vi "FPGA_Main_v7.vi"() -> ()   [LabVIEW 2018]
uses:
  <vilib>/Platform/TimedLoop/XDataNode/XDataNode.xnode
  <vilib>/Platform/TimedLoop/XDataNode/nitl_modes.ctl
  <vilib>/Platform/TimedLoop/XDataNode/XDNodeRunTimeDep.lvlib
  <vilib>/Platform/TimedLoop/XDataNode/wakeup.ctl
  <vilib>/Platform/TimedLoop/XDataNode/timing_clust.ctl
  <vilib>/rvi/DataTransferAndStorage/Container/XNode/niFpgaContainer.xnode
  <vilib>/rvi/FIFO/Fifo_Resource/nirvififoEmulationRead.vi
  <vilib>/eio/EIONode/EIONode.xnode
  <vilib>/rvi/eio/common/nirviEmuTemplateMethod_errors.vi
  <vilib>/rvi/DataTransferAndStorage/Register/Emulation/niFpgaRegisterEmulation.vi
  <instrlib>/_niInstr/Basic Elements/v1/FPGA/niInstr Basic Elements v1 FPGA.lvlib
  <vilib>/rvi/FIFO/Fifo_Resource/nirvififoEmulationWrite.vi
  <vilib>/rvi/interface/RandomDataEmulation/nirviRandomDataFpgaReadWriteTemplate.vi
  <instrlib>/_niInstr/Basic Elements/v1/FPGA/Private/Count Down U32.vi
  <instrlib>/_niInstr/Basic Elements/v1/FPGA/Private/Count Up U8.vi
  <vilib>/rvi/Memory/Memory_Emulation/nirvimemoryFastEmulation.vi
  <vilib>/rvi/Memory/Memory_Emulation/nirvimemoryEmulation.vi
  <vilib>/eio/EIOPropertyNode/EIOPropertyNode.xnode
  <vilib>/LabVIEW Targets/FPGA/RIO/BlueMoonOnboardIO/nicrio_cRIO-BlueMoonOnboardAi_TerminalMod.ctl
  <vilib>/rvi/eio/common/nirviEmuTemplatePropertyGet_errors.vi
  <vilib>/rvi/eio/common/nirviEmuTemplatePropertyGet_noerrors.vi
  <vilib>/rvi/eio/common/nirviEmuTemplatePropertySet_errors.vi
  <vilib>/rvi/eio/common/nirviEmuTemplatePropertySet_noerrors.vi
  <vilib>/LabVIEW Targets/FPGA/RIO/BlueMoonOnboardIO/nicrio_cRIO-BlueMoonOnboardAi_VoltageRange.ctl
  <instrlib>/_niInstr/Basic Elements/v1/FPGA/Private/Count Up U32.vi
panel:
  out "AuxArbWfm":u32
  in  "Reset":bool
  out "SubEventCode":u8
  out "Daq.Length?":u32
  in  "Start":bool
  out "RFU64 Ele#":u32
  out "EventCode Ele#":u32
  out "SigI16 Ele#":u32
  out "EventCode":u8
  out "DI":u8
  out "IonGateAGC.Time":u32
  out "IonGateAGC.Value":u64
  out "IonGateAGC.Target*TrialTime":u64
  out "Daq.AqNumber?":u32
  out "Daq.HighestValue_I16":i16
  out "AI.ReadingClocks":u32
  out "LaserTrig.Enable?":bool
  out "Event.Scan?":bool
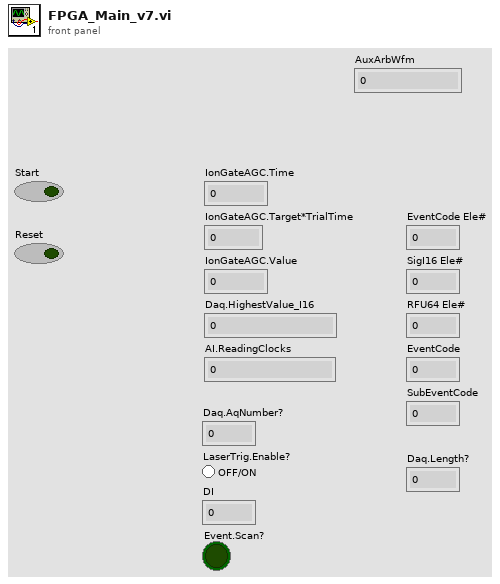
[diagram p1: front panel]
types:
  T1 = typedef "nicrio_cRIO-BlueMoonOnboardAi_VoltageRange.ctl" = u8
  T2 = typedef "nicrio_cRIO-BlueMoonOnboardAi_TerminalMod.ctl" = u8
  T3 = typedef "XDNodeRunTimeDep.lvlib/timing_clust.ctl" = cluster{"Expected End [f-1]":u64, "Actual End [f-1]":u64, "Finished Late? [f-1]":bool, "Expected End [i-1]":u64, "Actual End [i-1]":u64, "Finished Late? [i-1]":bool, "Expected Start [i]":u64, "Actual Start [i]":u64, "Expected Start [f]":u64, "Actual Start [f]":u64, "Source Name":string, "Structure Name":string, "Period":i64, "Deadline":i64, "Offset":i64, "Start":i64, "Priority":i32, "Timeout":i32, "Mode":T4, "Wakeup Reason":T5, "Error":errorcluster, "Source Type":string, "Secondary Source Type":string, "Global End Time":u64, "Global Start Time":u64, "Frame Duration":u64, "Iteration Duration":u64, "Assigned CPU":i32, "I/O Scan Engine Mode":u32}
  T4 = typedef "XDNodeRunTimeDep.lvlib/nitl_modes.ctl" = enum32{"No Change", "Process missed periods, maintain original phase", "Discard missed periods, maintain original phase", "Process missed periods, ignore original phase", "Discard missed periods, ignore original phase"}
  T5 = typedef "XDNodeRunTimeDep.lvlib/wakeup.ctl" = enum32{"Normal", "Aborted", "Asynchronous wakeup", "Timing source error", "Timed loop error", "Timeout"}
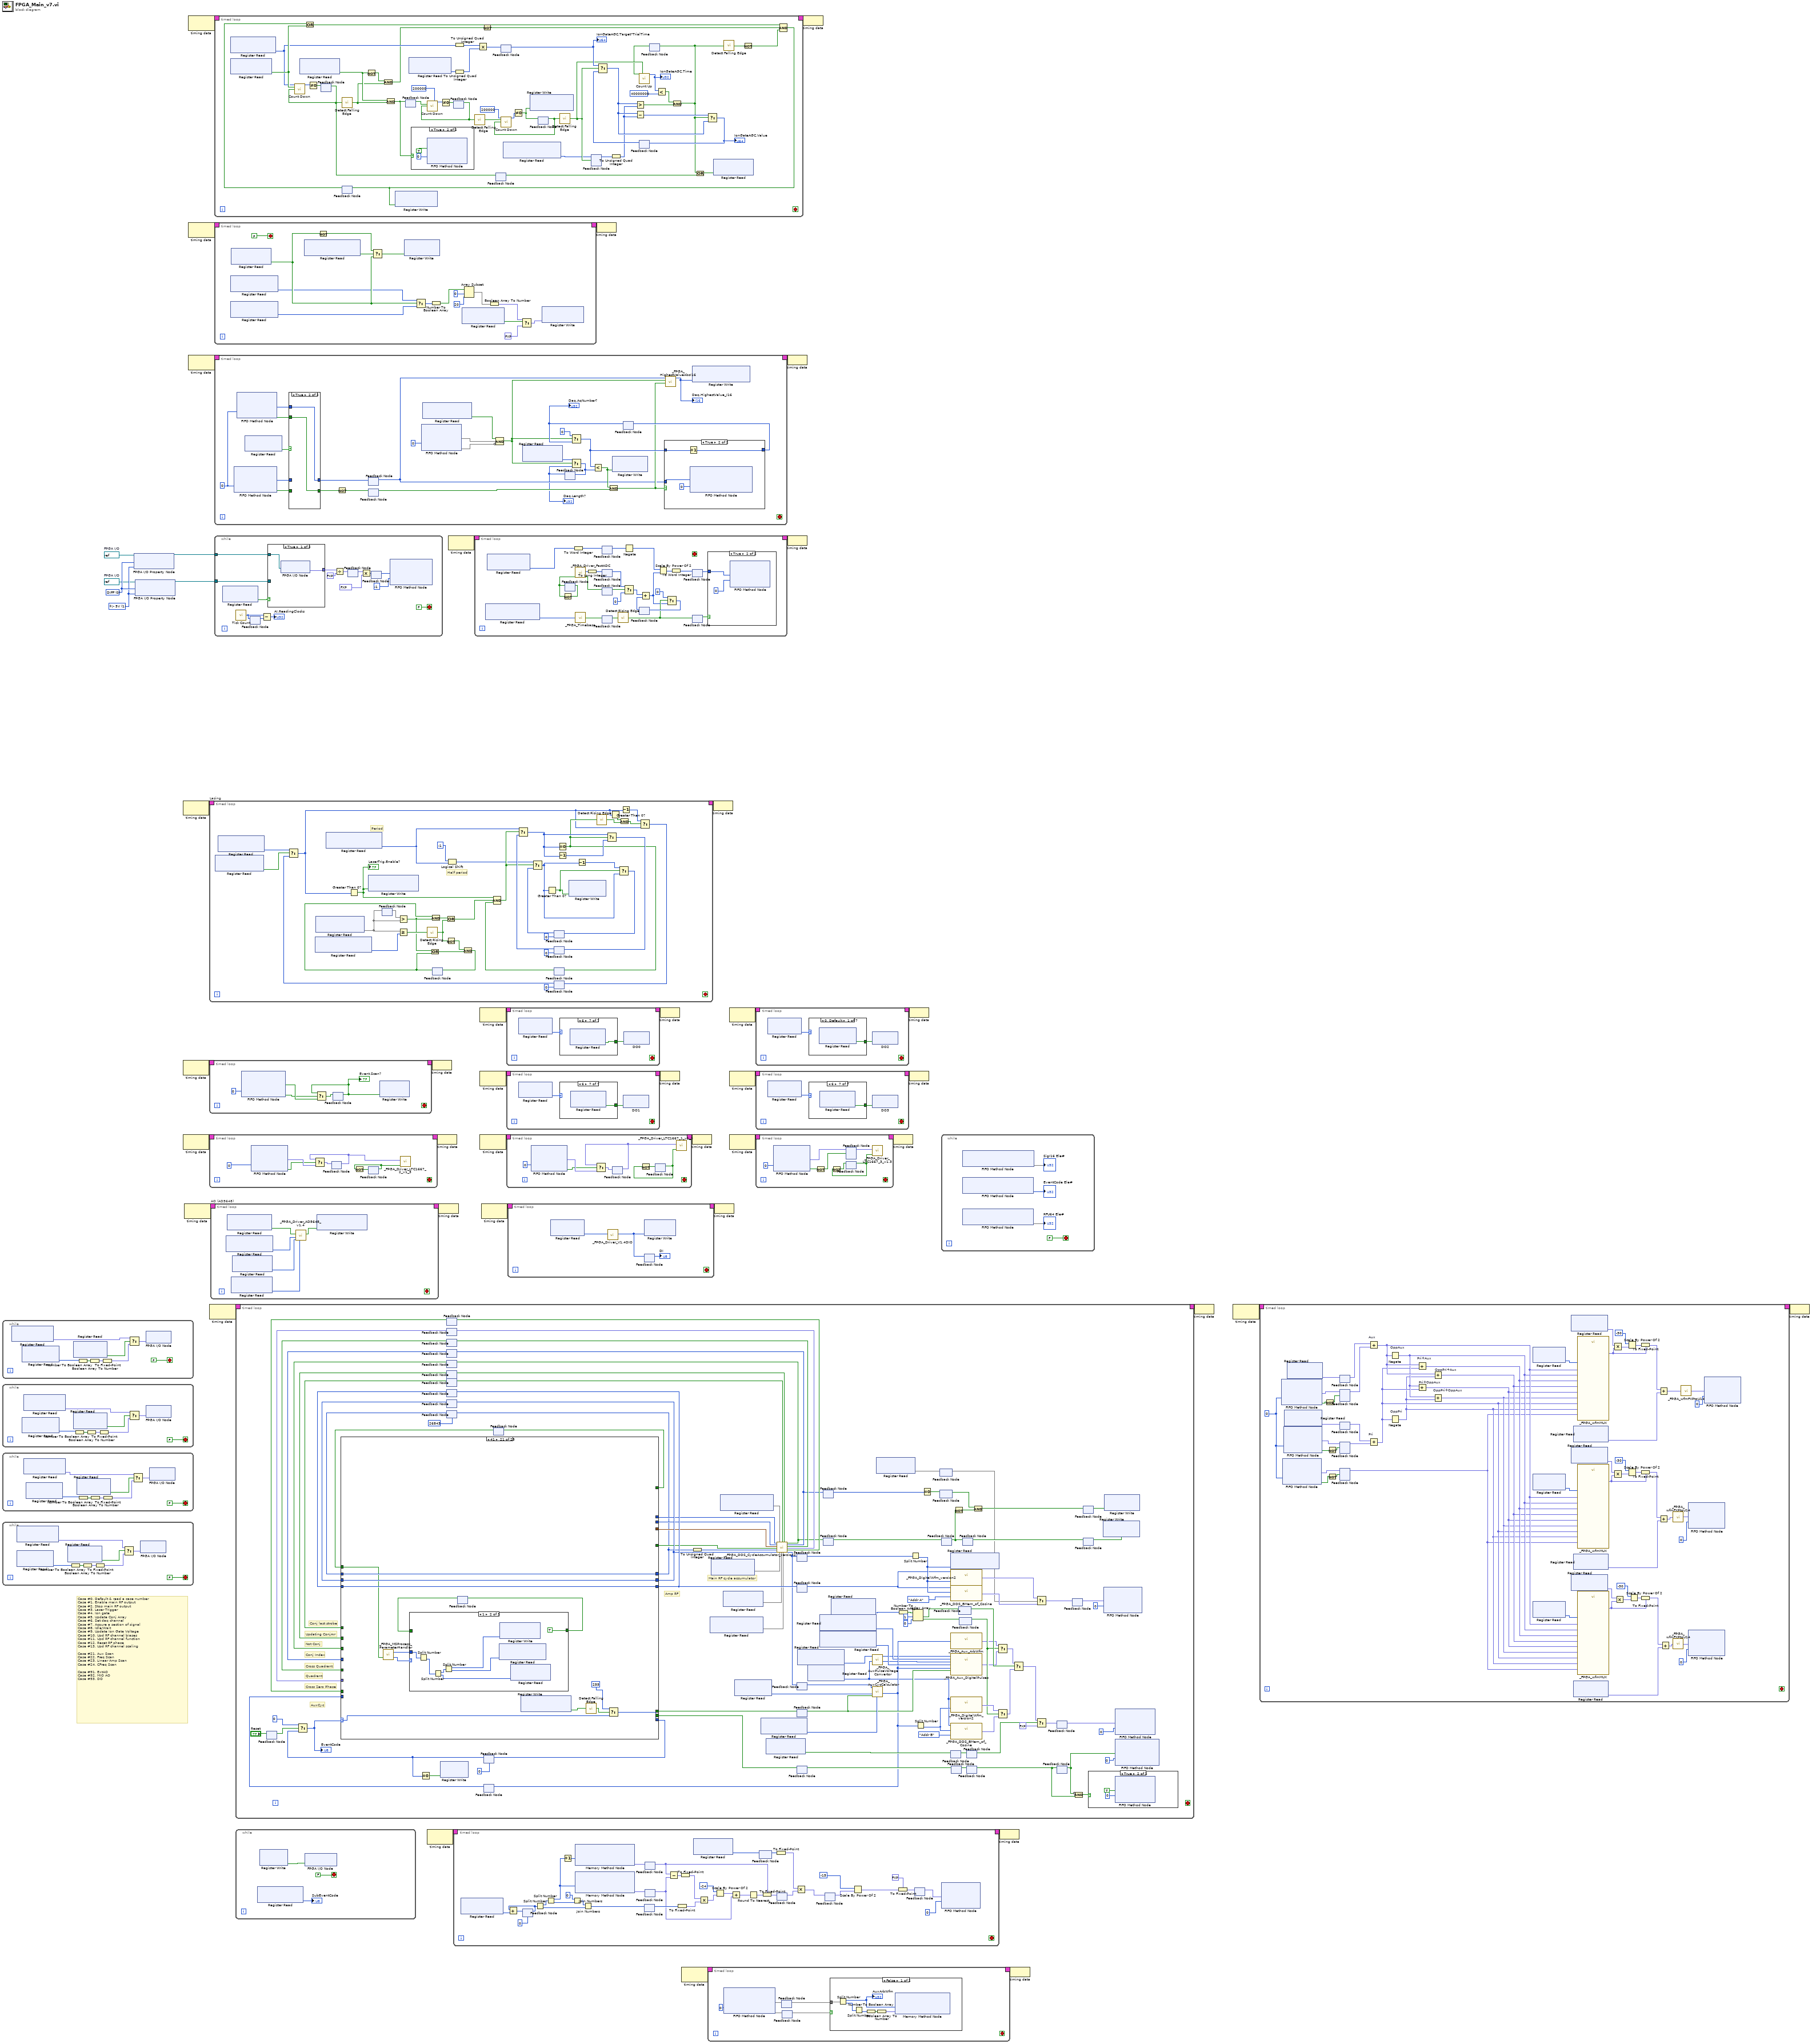
[diagram p0: block diagram]
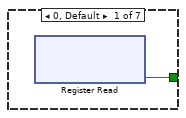
[diagram p3: hidden frame]
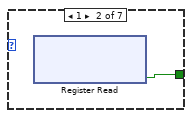
[diagram p4: hidden frame]
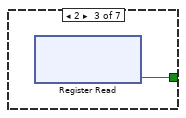
[diagram p5: hidden frame]
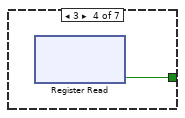
[diagram p6: hidden frame]
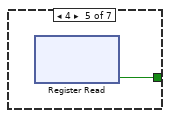
[diagram p7: hidden frame]
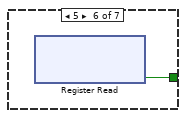
[diagram p8: hidden frame]
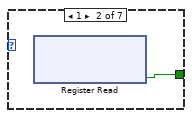
[diagram p9: hidden frame]
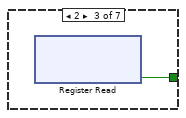
[diagram p10: hidden frame]
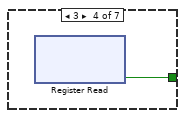
[diagram p11: hidden frame]
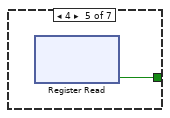
[diagram p12: hidden frame]
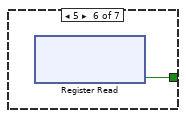
[diagram p13: hidden frame]
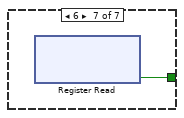
[diagram p14: hidden frame]
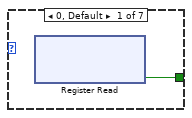
[diagram p15: hidden frame]
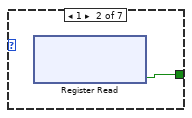
[diagram p16: hidden frame]
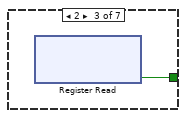
[diagram p17: hidden frame]
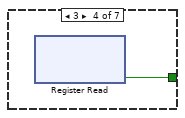
[diagram p18: hidden frame]
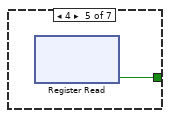
[diagram p19: hidden frame]
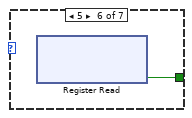
[diagram p20: hidden frame]
diagram:
  w4 = T1 1 items=["+/- 10V", "+/- 5V", "+/- 2V", "+/- 1V"] ("Voltage Range")
  w5 = T2 0 items=["DIFF", "RSE"] ("Terminal Mode")
  w1 = refnum<k21> "AI6"  # FPGA I/O
  w6 = refnum<k21> "AI7"  # FPGA I/O
  # "Case #0. Default & read a case number\nCase #1. Enable main RF output\nCase #2. Stop main RF output\nCase #3. Laser Trigger\nCase #4. Ion gate\nCase #5. Update Conj Array\nCase #6. Set daq channel\nCase #7. Acqure a section of signal\nCase #8. Idle/Wait\nCase #9. Update Ion Gate Voltage\nCase #10. Upd RF channel biases\nCase #11. Upd RF channel function\nCase #12. Reset RF phase\nCase #13. Upd RF channel scaling\n\nCase #21. Aux Scan\nCase #22. Freq Scan\nCase #23. Linear Amp Scan\nCase #24. CFreq Scan\n\nCase #91. ExtAO\nCase #92. MIO AO\nCase #93. DO"
  n1 = while {
    stop <- FALSE stop-if-true
    n2 = xnode ("Register Read")() -> ("Data"=w51:fxp<+/-,20,5>)  [unwired: 1 in, 1 out]
    n3 = xnode ("Register Read")() -> ("Data"=w47:u32)  [unwired: 1 in, 1 out]
    n4 = xnode ("Register Read")() -> ("Data"=w50:bool)  [unwired: 1 in, 1 out]
    n5 = Number To Boolean Array(number=w47) -> (Boolean array=w48:bool[])
    n6 = Boolean Array To Number(Boolean array=w48) -> (number=w49:fxp<+/-,32,5>)
    n7 = To Fixed-Point(number=w49) -> (fixed-point=w46:fxp<+/-,20,5>)  [unwired: 1 in]
    n8 = Select(t=w51, s=w50, f=w46) -> (s? t:f=w52:fxp<+/-,20,5>)
    n9 = xnode "FPGA I/O Node"("AO0"=w52) -> ()  [unwired: 1 in, 1 out]
  }
  n10 = while {
    stop <- FALSE stop-if-true
    n11 = xnode ("Register Read")() -> ("Data"=w59:u32)  [unwired: 1 in, 1 out]
    n12 = xnode ("Register Read")() -> ("Data"=w54:fxp<+/-,20,5>)  [unwired: 1 in, 1 out]
    n13 = xnode ("Register Read")() -> ("Data"=w56:bool)  [unwired: 1 in, 1 out]
    n14 = Number To Boolean Array(number=w59) -> (Boolean array=w57:bool[])
    n15 = Boolean Array To Number(Boolean array=w57) -> (number=w58:fxp<+/-,32,5>)
    n16 = To Fixed-Point(number=w58) -> (fixed-point=w60:fxp<+/-,20,5>)  [unwired: 1 in]
    n17 = Select(t=w54, s=w56, f=w60) -> (s? t:f=w55:fxp<+/-,20,5>)
    n18 = xnode "FPGA I/O Node"("AO1"=w55) -> ()  [unwired: 1 in, 1 out]
  }
  n19 = while {
    stop <- FALSE stop-if-true
    n20 = xnode ("Register Read")() -> ("Data"=w62:fxp<+/-,20,5>)  [unwired: 1 in, 1 out]
    n21 = xnode ("Register Read")() -> ("Data"=w67:u32)  [unwired: 1 in, 1 out]
    n22 = xnode ("Register Read")() -> ("Data"=w64:bool)  [unwired: 1 in, 1 out]
    n23 = Number To Boolean Array(number=w67) -> (Boolean array=w66:bool[])
    n24 = Boolean Array To Number(Boolean array=w66) -> (number=w65:fxp<+/-,32,5>)
    n25 = To Fixed-Point(number=w65) -> (fixed-point=w68:fxp<+/-,20,5>)  [unwired: 1 in]
    n26 = Select(t=w62, s=w64, f=w68) -> (s? t:f=w63:fxp<+/-,20,5>)
    n27 = xnode "FPGA I/O Node"("AO2"=w63) -> ()  [unwired: 1 in, 1 out]
  }
  n28 = while {
    stop <- FALSE stop-if-true
    n29 = xnode ("Register Read")() -> ("Data"=w70:fxp<+/-,20,5>)  [unwired: 1 in, 1 out]
    n30 = xnode ("Register Read")() -> ("Data"=w75:u32)  [unwired: 1 in, 1 out]
    n31 = xnode ("Register Read")() -> ("Data"=w72:bool)  [unwired: 1 in, 1 out]
    n32 = Number To Boolean Array(number=w75) -> (Boolean array=w73:bool[])
    n33 = Boolean Array To Number(Boolean array=w73) -> (number=w74:fxp<+/-,32,5>)
    n34 = To Fixed-Point(number=w74) -> (fixed-point=w76:fxp<+/-,20,5>)  [unwired: 1 in]
    n35 = Select(t=w70, s=w72, f=w76) -> (s? t:f=w71:fxp<+/-,20,5>)
    n36 = xnode "FPGA I/O Node"("AO3"=w71) -> ()  [unwired: 1 in, 1 out]
  }
  n37 = xnode "FPGA I/O Property Node"("FPGA I/O In"=w6, "Terminal Mode"=w5, "Voltage Range"=w4) -> ("FPGA I/O Out"=w3:refnum<k21>)
  n38 = xnode "FPGA I/O Property Node"("FPGA I/O In"=w1, "Terminal Mode"=w5, "Voltage Range"=w4) -> ("FPGA I/O Out"=w2:refnum<k21>)
  n39 = node-c288() -> (w38:T3)  [unwired: 1 in]
  n40 = node-c288() -> (w16:T3)  [unwired: 1 in]
  n41 = node-c288() -> (w40:T3)  [unwired: 1 in]
  n42 = node-c288() -> (w44:T3)  [unwired: 1 in]
  n43 = node-c288() -> (w34:T3)  [unwired: 1 in]
  n44 = node-c288() -> (w28:T3)  [unwired: 1 in]
  n45 = node-c288() -> (w36:T3)  [unwired: 1 in]
  n46 = timed-loop "Lasing" {
    timing: w38 -> [_]
    timing-out: [_] -> w37
    stop <- _ stop-if-true
    # "Half period"
    # "Period"
    n47 = xnode ("Register Read")() -> ("Data"=w91:bool)  [unwired: 1 in, 1 out]
    n48 = xnode ("Register Read")() -> ("Data"=w101:u8)  [unwired: 1 in, 1 out]
    n49 = xnode ("Register Read")() -> ("Data"=w102:u32)  [unwired: 1 in, 1 out]
    n50 = xnode ("Register Read")() -> ("Data"=w90)  [unwired: 1 in, 1 out]
    n51 = xnode ("Register Read")() -> ("Data"=w103:u32)  [unwired: 1 in, 1 out]
    n52 = feedback-in #1(w90) -> ()
    n53 = feedback #1() -> (w98)  [unwired: 1 in]
    n54 = Greater?(x=w98, y=w90) -> (0:w92:bool)
    n55 = Greater Or Equal?(x=w90, y=w102) -> (x >= y?=w115:bool)
    n56 = call <instrlib>:"Detect Rising Edge.vi"("signal"=w115) -> ("edge detected"=w97:bool)  [unwired: 14 in]
    n57 = feedback #2() -> (w94:bool)  [unwired: 1 in]
    n58 = Or(x=w92, y=w94) -> (x .or. y?=w93:bool)
    n59 = And(x=w94, y=w92) -> (x .and. y?=w95:bool)
    n60 = Or(x=w95, y=w97) -> (x .or. y?=w96:bool)
    n61 = Not(x=w97) -> (.not. x?=w100:bool)
    n62 = Logical Shift(y=i16 -1 ("n"), x=w103) -> (x << y=w112:u32)
    n63 = And(x=w100, y=w93) -> (x .and. y?=w99:bool)
    n64 = feedback-in #2(w99) -> ()
    n65 = feedback #3(u32 0) -> (w108:u32)
    n66 = feedback #4(u32 0 ("Data")) -> (w116:u32)
    n67 = feedback #5() -> (w89:bool)  [unwired: 1 in]
    n68 = feedback #6(u8 0 ("f")) -> (w104:u8)
    n69 = Select(t=w101, s=w91, f=w104) -> (s? t:f=w81:u8)
    n70 = Greater Than 0?(x=w81) -> (x > 0?=w78:bool)
    "LaserTrig.Enable?" <- w78
    n71 = xnode ("Register Write")("Data"=w78) -> ()  [unwired: 1 in, 1 out]
    n72 = Compound Arithmetic op=AND(w78, w96, w89) -> (w113:bool)
    n73 = Select(t=w103, s=w113, f=w116) -> (s? t:f=w87:u32)
    n74 = Select(t=w112, s=w113, f=w108) -> (s? t:f=w110:u32)
    n75 = Greater Than 0?(x=w110) -> (x > 0?=w77:bool)
    n76 = Equal To 0?(x=w87) -> (x = 0?=w83:bool)
    n77 = feedback-in #5(w83) -> ()
    n78 = Decrement(x=w87) -> (x-1=w88:u32)
    n79 = xnode ("Register Write")("Data"=w77) -> ()  [unwired: 1 in, 1 out]
    n80 = Decrement(x=w110) -> (x-1=w111:u32)
    n81 = call <instrlib>:"Detect Rising Edge.vi"("signal"=w83) -> ("edge detected"=w82:bool)  [unwired: 14 in]
    n82 = Select(t=w87, s=w83, f=w88) -> (s? t:f=w107:u32)
    n83 = feedback-in #4(w107) -> ()
    n84 = Greater Than 0?(x=w81) -> (x > 0?=w79:bool)
    n85 = Select(t=w111, s=w77, f=w110) -> (s? t:f=w109:u32)
    n86 = feedback-in #3(w109) -> ()
    n87 = And(x=w79, y=w82) -> (x .and. y?=w80:bool)
    n88 = Decrement(x=w81) -> (x-1=w106:u8)
    n89 = Select(t=w106, s=w80, f=w81) -> (s? t:f=w105:u8)
    n90 = feedback-in #6(w105) -> ()
  }
  n91 = timed-loop {
    timing: w16 -> [_]
    timing-out: [_] -> w15
    stop <- _ stop-if-true
    n92 = xnode ("FIFO Method Node")("Timeout"=0) -> ("Element"=w122:bool, "Timed Out?"=w121:bool)  [unwired: 1 in, 1 out]
    n93 = feedback #7() -> (w123:bool)  [unwired: 1 in]
    "Event.Scan?" <- w123
    n94 = Select(t=w123, s=w121, f=w122) -> (s? t:f=w120:bool)
    n95 = feedback-in #7(w120) -> ()
    n96 = xnode ("Register Write")("Data"=w123) -> ()  [unwired: 1 in, 1 out]
  }
  n97 = timed-loop {
    timing: w40 -> [_]
    timing-out: [_] -> w39
    stop <- _ stop-if-true
    n98 = xnode ("FIFO Method Node")("Timeout"=0) -> ("Element"=w128:fxp<+,14,14>, "Timed Out?"=w126:bool)  [unwired: 1 in, 1 out]
    n99 = feedback #8() -> (w129:fxp<+,14,14>)  [unwired: 1 in]
    n100 = Select(t=w129, s=w126, f=w128) -> (s? t:f=w130:fxp<+,14,14>)
    n101 = feedback-in #8(w130) -> ()
    n102 = feedback #9() -> (w131:bool)  [unwired: 1 in]
    n103 = Not(x=w131) -> (.not. x?=w132:bool)
    n104 = feedback-in #9(w132) -> ()
    n105 = call "_FPGA_Driver_LTC1667_2_v1_3.vi"("Clk"=w131, "Data in"=w129) -> ()  [unwired: 10 in]
  }
  n106 = node-c288() -> (w42:T3)  [unwired: 1 in]
  n107 = timed-loop "AO (AD5648)" {
    timing: w44 -> [_]
    timing-out: [_] -> w43
    stop <- _ stop-if-true
    n108 = xnode ("Register Read")() -> ("Data"=w137:u8)  [unwired: 1 in, 1 out]
    n109 = xnode ("Register Read")() -> ("Data"=w138:bool)  [unwired: 1 in, 1 out]
    n110 = xnode ("Register Read")() -> ("Data"=w135:u8)  [unwired: 1 in, 1 out]
    n111 = xnode ("Register Read")() -> ("Data"=w136:u16)  [unwired: 1 in, 1 out]
    n112 = call "_FPGA_Driver_AD5648_v1.4.vi"("Cmd#"=w135, "AO Data"=w136, "Channel#"=w137, "Update_latch"=w138) -> ("Updating?"=w139:bool)  [unwired: 7 in]
    n113 = xnode ("Register Write")("Data"=w139) -> ()  [unwired: 1 in, 1 out]
  }
  n114 = timed-loop {
    timing: w34 -> [_]
    timing-out: [_] -> w33
    stop <- _ stop-if-true
    n115 = xnode ("Register Read")() -> ("Data"=w170:u32)  [unwired: 1 in, 1 out]
    n116 = xnode ("Register Read")() -> ("Data"=w173:bool)  [unwired: 1 in, 1 out]
    n117 = xnode ("Register Read")() -> ("Data"=w149:bool)  [unwired: 1 in, 1 out]
    n118 = feedback #10() -> (w172:bool)  [unwired: 1 in]
    n119 = call-poly <instrlib>:"Count Down.vi"("count in"=w170, "load"=w173, "decrement"=w172) -> ("count out"=w174:u32)  [unwired: 11 in, 1 out]
    n120 = Not Equal To 0?(x=w174) -> (x != 0?=w175:bool)
    n121 = feedback-in #10(w175) -> ()
    n122 = call <instrlib>:"Detect Falling Edge.vi"("signal"=w172) -> ("edge detected"=w147:bool)  [unwired: 14 in]
    n123 = feedback #11() -> (w188:bool)  [unwired: 1 in]
    n124 = Or(x=w188, y=w173) -> (x .or. y?=w146:bool)
    n125 = Not(x=w149) -> (.not. x?=w148:bool)
    n126 = And(x=w148, y=w147) -> (x .and. y?=w144:bool)
    n127 = And(x=w149, y=w147) -> (x .and. y?=w142:bool)
    n128 = feedback #12() -> (w179:bool)  [unwired: 1 in]
    n129 = feedback-in #12(w142) -> ()
    n130 = xnode ("Register Read")() -> ("Data"=w171:u32)  [unwired: 1 in, 1 out]
    n131 = case shown="True" w142 {
      frame False {
      }
      frame True {
        n132 = xnode ("FIFO Method Node")("Element"=TRUE, "Timeout"=0) -> ()  [unwired: 1 in, 2 out]
      }
    }
    n133 = feedback #13() -> (w177:bool)  [unwired: 1 in]
    n134 = call-poly <instrlib>:"Count Down.vi"("count in"=u32 200000, "load"=w179, "decrement"=w177) -> ("count out"=w181:u32)  [unwired: 11 in, 1 out]
    n135 = Not Equal To 0?(x=w181) -> (x != 0?=w178:bool)
    n136 = feedback-in #13(w178) -> ()
    n137 = To Unsigned Quad Integer(1:w170) -> (0:w167:u64)
    n138 = To Unsigned Quad Integer(1:w171) -> (0:w166:u64)
    n139 = call <instrlib>:"Detect Falling Edge.vi"("signal"=w177) -> ("edge detected"=w176:bool)  [unwired: 14 in]
    n140 = Multiply(x=w167, y=w166) -> (x*y=w168:u64)
    n141 = Not(x=w144) -> (.not. x?=w143:bool)
    n142 = feedback-in #14(w172) -> ()
    n143 = feedback #14() -> (w183:bool)  [unwired: 1 in]
    n144 = feedback-in #15(w168) -> ()
    n145 = feedback #15() -> (w165:u64)  [unwired: 1 in]
    "IonGateAGC.Target*TrialTime" <- w165
    n146 = xnode ("Register Read")() -> ("Data"=w161:i16)  [unwired: 1 in, 1 out]
    n147 = feedback #16() -> (w169:bool)  [unwired: 1 in]
    n148 = call-poly <instrlib>:"Count Down.vi"("count in"=u32 200000, "load"=w176, "decrement"=w169) -> ("count out"=w184:u32)  [unwired: 11 in, 1 out]
    n149 = Not Equal To 0?(x=w184) -> (x != 0?=w180:bool)
    n150 = xnode ("Register Write")("Data"=w180) -> ()  [unwired: 1 in, 1 out]
    n151 = feedback-in #16(w180) -> ()
    n152 = call <instrlib>:"Detect Falling Edge.vi"("signal"=w169) -> ("edge detected"=w162:bool)  [unwired: 14 in]
    n153 = feedback #17() -> (w160:i16)  [unwired: 1 in]
    n154 = feedback-in #17(w161, w162) -> ()
    n155 = To Unsigned Quad Integer(1:w160) -> (0:w153:u64)
    n156 = feedback #18() -> (w163:u64)  [unwired: 1 in]
    n157 = Select(t=w165, s=w162, f=w163) -> (s? t:f=w154:u64)
    n158 = Greater?(x=w154, y=w153) -> (0:w152:bool)
    n159 = Subtract(x=w154, y=w153) -> (x-y=w164:u64)
    n160 = feedback #19() -> (w151:bool)  [unwired: 1 in]
    n161 = call-poly <instrlib>:"Count Up.vi"("increment"=w151, "reset"=w162) -> ("count out"=w158:u32)  [unwired: 13 in]
    "IonGateAGC.Time" <- w158
    n162 = Less?(x=w158, y=u32 40000000) -> (x < y?=w156:bool)
    n163 = And(x=w156, y=w152) -> (x .and. y?=w150:bool)
    n164 = feedback-in #19(w150) -> ()
    n165 = Or(x=w150, y=w183) -> (x .or. y?=w187:bool)
    n166 = Select(t=w164, s=w150, f=w154) -> (s? t:f=w155:u64)
    "IonGateAGC.Value" <- w155
    n167 = feedback-in #18(w155) -> ()
    n168 = xnode ("Register Read")("Data"=w187) -> ()  [unwired: 1 in, 1 out]
    n169 = call <instrlib>:"Detect Falling Edge.vi"("signal"=w150) -> ("edge detected"=w159:bool)  [unwired: 14 in]
    n170 = Not(x=w159) -> (.not. x?=w145:bool)
    n171 = Compound Arithmetic op=AND(w146, w143, w145) -> (w185:bool)
    n172 = feedback-in #11(w185) -> ()
    n173 = xnode ("Register Write")("Data"=w185) -> ()  [unwired: 1 in, 1 out]
  }
  n174 = timed-loop {
    timing: w28 -> [_]
    timing-out: [_] -> w27
    stop <- FALSE stop-if-true
    n175 = xnode ("Register Read")() -> ("Data"=w202:u32)  [unwired: 1 in, 1 out]
    n176 = xnode ("Register Read")() -> ("Data"=w203:u32)  [unwired: 1 in, 1 out]
    n177 = xnode ("Register Read")() -> ("Data"=w205:bool)  [unwired: 1 in, 1 out]
    n178 = xnode ("Register Read")() -> ("Data"=w206:bool)  [unwired: 1 in, 1 out]
    n179 = Not(x=w205) -> (.not. x?=w204:bool)
    n180 = Select(t=w204, s=w206, f=w205) -> (s? t:f=w193:bool)
    n181 = xnode ("Register Write")("Data"=w193) -> ()  [unwired: 1 in, 1 out]
    n182 = Select(t=w202, s=w205, f=w203) -> (s? t:f=w200:u32)
    n183 = Number To Boolean Array(number=w200) -> (Boolean array=w198:bool[])
    n184 = xnode ("Register Read")() -> ("Data"=w207:bool)  [unwired: 1 in, 1 out]
    n185 = Array Subset(array=w198, index=0, length=20) -> (w195:bool[])
    n186 = Boolean Array To Number(Boolean array=w195) -> (number=w194:fxp<+/-,20,5>)
    n187 = Select(t=w194, s=w207, f=fxp<+/-,20,5> 0.0) -> (s? t:f=w201:fxp<+/-,20,5>)
    n188 = xnode ("Register Write")("Data"=w201) -> ()  [unwired: 1 in, 1 out]
  }
  n189 = timed-loop {
    timing: w36 -> [_]
    timing-out: [_] -> w35
    stop <- _ stop-if-true
    w224 = 0 ("Timeout")
    n190 = xnode ("FIFO Method Node")("Timeout"=w224) -> ("Element"=w225:i16, "Timed Out?"=w226:bool)  [unwired: 1 in, 1 out]
    n191 = xnode ("FIFO Method Node")("Timeout"=w224) -> ("Element"=w228:i16, "Timed Out?"=w227:bool)  [unwired: 1 in, 1 out]
    n192 = xnode ("Register Read")() -> ("Data"=w229:bool)  [unwired: 1 in, 1 out]
    n193 = case shown="True" w229 {
      tunnel: w228 -> [_ w240]
      tunnel: w227 -> [_ w239]
      tunnel: w226 -> [w237 _]
      tunnel: w225 -> [w238 _]
      tunnel: [w238 w240] -> w217
      tunnel: [w237 w239] -> w220
      frame False {
      }
      frame True {
      }
    }
    n194 = Not(x=w220) -> (.not. x?=w213:bool)
    n195 = feedback #20() -> (w222:i16)  [unwired: 1 in]
    n196 = feedback-in #20(w217) -> ()
    n197 = feedback-in #21(w213) -> ()
    n198 = feedback #21() -> (w221:bool)  [unwired: 1 in]
    n199 = xnode ("FIFO Method Node")("Timeout"=0) -> ("Element"=w215, "Timed Out?"=w212)  [unwired: 1 in, 1 out]
    n200 = xnode ("Register Read")() -> ("Data"=w211:bool)  [unwired: 1 in, 1 out]
    n201 = Compound Arithmetic op=AND(w211, w215, invert w212) -> (w214:bool)
    n202 = xnode ("Register Read")() -> ("Data"=w232:u32)  [unwired: 1 in, 1 out]
    n203 = feedback #22() -> (w218:u32)  [unwired: 1 in]
    "Daq.Length?" <- w218
    n204 = Select(t=w232, s=w214, f=w218) -> (s? t:f=w230:u32)
    n205 = feedback-in #22(w230) -> ()
    n206 = feedback #23() -> (w219:u32)  [unwired: 1 in]
    "Daq.AqNumber?" <- w219
    n207 = Select(t=u32 0, s=w214, f=w219) -> (s? t:f=w236:u32)
    n208 = Less?(x=w236, y=w230) -> (x < y?=w233:bool)
    n209 = And(x=w233, y=w221) -> (x .and. y?=w223:bool)
    n210 = xnode ("Register Write")("Data"=w233) -> ()  [unwired: 1 in, 1 out]
    n211 = case shown="True" w223 {
      tunnel: [w241 w243] -> w231
      tunnel: w236 -> [w241 w244]
      tunnel: w222 -> [_ w242]
      frame False {
      }
      frame True {
        n212 = Increment(x=w244) -> (x+1=w243:u32)
        n213 = xnode ("FIFO Method Node")("Element"=w242, "Timeout"=0) -> ()  [unwired: 1 in, 2 out]
      }
    }
    n214 = feedback-in #23(w231) -> ()
    n215 = call "_FPGA_HighestValueAbsI16.vi"("Enable"=w223, "Init"=w214, "Value in"=w222) -> ("Highest Value"=w234:i16)  [unwired: 8 in]
    "Daq.HighestValue_I16" <- w234
    n216 = xnode ("Register Write")("Data"=w234) -> ()  [unwired: 1 in, 1 out]
  }
  n217 = while {
    tunnel: w3 -> [w249]
    tunnel: w2 -> [w248]
    stop <- FALSE stop-if-true
    n218 = xnode ("Register Read")() -> ("Data"=w250:bool)  [unwired: 1 in, 1 out]
    n219 = call "Tick Count"() -> ("Tick Count(Ticks)"=w260:u32)
    n220 = feedback #24() -> (w261:u32)  [unwired: 1 in]
    n221 = feedback-in #24(w260) -> ()
    n222 = Subtract(x=w260, y=w261) -> (x-y=→"AI.ReadingClocks":u32)
    n223 = case shown="True" w250 {
      tunnel: [w264 w266] -> w251
      tunnel: w249 -> [w263 _]
      tunnel: w248 -> [_ w265]
      frame True {
        n224 = xnode "FPGA I/O Node"("FPGA I/O In"=w263) -> ("I/O Item"=w264:fxp<+/-,24,5>)  [unwired: 1 out]
      }
      frame False {
        n225 = xnode "FPGA I/O Node"("FPGA I/O In"=w265) -> ("I/O Item"=w266:fxp<+/-,24,5>)  [unwired: 1 out]
      }
    }
    n226 = Divide(x=w251, y=fxp<+,3,3> 5.0) -> (x/y=w254:fxp<+/-,24,1>)
    n227 = feedback #25() -> (w257:fxp<+/-,24,1>)  [unwired: 1 in]
    n228 = feedback-in #25(w254) -> ()
    n229 = Multiply(x=w257, y=fxp<+,15,15> 32767.0) -> (x*y=w256:i16)
    n230 = feedback #26() -> (w252:i16)  [unwired: 1 in]
    n231 = feedback-in #26(w256) -> ()
    n232 = xnode ("FIFO Method Node")("Element"=w252, "Timeout"=-1) -> ()  [unwired: 1 in, 2 out]
  }
  n233 = timed-loop {
    timing: w42 -> [_]
    timing-out: [_] -> w41
    stop <- _ stop-if-true
    # "Amp RF"
    # "AuxCyc"
    # "Conj last strobe"
    # "Main RF cycle accumulator"
    # "Cross Zero Phase"
    # "Quadrant"
    # "Cross Quadrant"
    # "Conj Index"
    # "Not Conj"
    # "Updating ConjArr"
    n234 = feedback-in #27("Reset") -> ()
    n235 = feedback #27() -> (w300:bool)  [unwired: 1 in]
    n236 = feedback #28() -> (w355:bool)  [unwired: 1 in]
    n237 = feedback #29() -> (w267:fxp<+,2,2>)  [unwired: 1 in]
    n238 = feedback #30() -> (w356:bool)  [unwired: 1 in]
    n239 = feedback #31() -> (w362:u8)  [unwired: 1 in]
    n240 = feedback #32() -> (w363:bool)  [unwired: 1 in]
    n241 = feedback #33() -> (w359:bool)  [unwired: 1 in]
    n242 = feedback #34() -> (w302:bool)  [unwired: 1 in]
    n243 = feedback #35() -> (w369:u32)  [unwired: 1 in]
    n244 = feedback #36() -> (w368:u32)  [unwired: 1 in]
    n245 = feedback #37(u32 26843) -> (w367:u32)
    n246 = feedback #38(u8 0 ("t")) -> (w299:u8)
    n247 = Select(t=u8 0, s=w300, f=w299) -> (s? t:f=w297:u8)
    "EventCode" <- w297
    n248 = Equal To 0?(x=w299) -> (x = 0?=w327:bool)
    n249 = xnode ("Register Write")("Data"=w327) -> ()  [unwired: 1 in, 1 out]
    n250 = feedback #39() -> (w333:u64)  [unwired: 1 in]
    n251 = feedback #40() -> (w345:bool)  [unwired: 1 in]
    n252 = case shown="41" w297 {
      selector: w297 -> [_ w414 w443 w514 w525 w556 w590 w657 w685 w716 w759 w778 w797 w814 w837 w856 w892 w977 w1111 w1327 w1390 w1412 w1458 w1473 w1502]
      tunnel: [w401 w431 w442 w513 w522 w555 w589 w656 w684 w715 w758 w777 w796 w813 w836 w855 w891 w976 w1110 w1326 w1393 w1411 w1457 w1472 w1501] -> w371
      tunnel: [w400 w430 w450 w510 w530 w559 w596 w654 w682 w709 w760 w779 w798 w815 w838 w860 w881 w985 w1106 w1315 w1402 w1418 w1464 w1479 w1508] -> w320
      tunnel: [w399 w429 w449 w509 w529 w560 w595 w653 w681 w708 w761 w780 w799 w816 w839 w861 w880 w984 w1105 w1334 w1401 w1417 w1463 w1478 w1507] -> w364
      tunnel: [w398 w428 w448 w516 w528 w561 w594 w652 w680 w707 w762 w781 w800 w817 w840 w862 w879 w983 w1115 w1333 w1400 w1416 w1462 w1477 w1506] -> w366
      tunnel: w369 -> [w398 w428 w445 w515 w528 w561 w594 w652 w680 w707 w762 w781 w800 w817 w840 w862 w879 w980 w1114 w1330 w1400 w1416 w1462 w1477 w1506]
      tunnel: w368 -> [w399 w429 w446 w509 w529 w560 w595 w653 w681 w708 w761 w780 w799 w816 w839 w861 w880 w981 w1105 w1331 w1401 w1417 w1463 w1478 w1507]
      tunnel: w367 -> [w400 w430 w447 w510 w530 w559 w596 w654 w682 w709 w760 w779 w798 w815 w838 w860 w881 w982 w1106 w1332 w1402 w1418 w1464 w1479 w1508]
      tunnel: w363 -> [_ _ _ _ _ _ w588 _ _ _ _ _ _ _ _ _ _ _ _ _ _ _ _ _ _]
      tunnel: w362 -> [_ _ w440 _ _ _ _ _ _ _ _ _ _ _ _ _ w876 w968 w1090 w1318 _ _ _ _ _]
      tunnel: w359 -> [_ _ _ _ _ _ w586 _ _ _ _ _ _ _ _ _ _ _ _ _ _ _ _ _ _]
      tunnel: w356 -> [_ _ _ _ _ _ _ _ _ _ _ _ _ _ _ _ _ _ w1086 _ _ _ _ _ _]
      tunnel: w267 -> [_ _ _ _ _ _ _ _ _ _ _ _ _ _ _ _ _ _ w1081 _ _ _ _ _ _]
      tunnel: w355 -> [_ _ _ _ _ _ _ _ _ _ _ _ _ _ _ _ _ _ _ _ _ _ _ _ _]
      tunnel: [_ _ _ _ _ _ w600 _ _ _ _ _ _ _ _ _ _ _ _ _ _ _ _ _ _] -> w350
      tunnel: [_ _ _ _ _ _ w599 _ _ _ _ _ _ _ _ _ _ _ _ _ _ _ _ _ _] -> w349
      tunnel: [_ _ _ _ _ _ w598 _ _ _ _ _ _ _ _ _ _ _ _ _ _ _ _ _ _] -> w348
      tunnel: [_ _ _ _ _ _ w591 _ _ _ _ _ _ _ _ _ _ _ _ _ _ _ _ _ _] -> w347
      tunnel: [TRUE TRUE _ _ _ _ _ _ _ _ _ _ _ _ _ _ _ _ _ _ _ _ _ _ _] -> w346
      tunnel: w345 -> [_ w410 w441 w511 w531 w562 w597 w655 w683 w714 w763 w782 w801 w818 w841 w852 w890 w975 w1109 w1325 w1399 w1415 w1461 w1476 w1505]
      tunnel: [_ _ _ _ _ _ _ _ _ _ _ _ _ _ _ _ w886 w973 w1104 _ _ _ _ _ _] -> w307
      tunnel: w333 -> [_ _ _ _ _ _ _ _ _ _ _ _ _ _ _ _ w885 w972 w1108 w1321 _ _ _ _ _]
      tunnel: [_ _ _ _ _ _ _ _ _ _ _ _ _ _ _ _ w882 w969 w1107 w1308 _ _ _ _ _] -> w332
      tunnel: w302 -> [_ _ w434 _ _ _ _ _ _ _ _ _ _ _ _ _ w872 w964 w1084 w1316 _ _ _ _ _]
      frame 0, Default {
        w375 = u32 536870912  # 2^29
        n253 = feedback-in #41("Start") -> ()
        n254 = feedback #41(FALSE ("Start")) -> (w378:bool)
        n255 = feedback #42() -> (w377:bool)  [unwired: 1 in]
        n256 = Or(x=w377, y=w378) -> (x .or. y?=w380:bool)
        n257 = feedback #43() -> (w381:bool)  [unwired: 1 in]
        n258 = Not(x=w381) -> (.not. x?=w376:bool)
        n259 = And(x=w380, y=w376) -> (x .and. y?=w379:bool)
        n260 = feedback-in #42(w379) -> ()
        n261 = call "_FPGA_MSProcess_DataReader.vi"("Read"=w379) -> ("Element"=w392:u64, "new data"=w382:bool)
        n262 = feedback-in #43(w382) -> ()
        n263 = Split Number(x=w392) -> (hi(x)=w388:u32, lo(x)=w390:u32)
        n264 = xnode ("Register Write")("Data"=FALSE) -> ()  [unwired: 1 in, 1 out]
        n265 = Split Number(x=w388) -> (lo(x)=w391:u16)  [unwired: 1 out]
        n266 = xnode ("Register Write")("Data"=w375) -> ()  [unwired: 1 in, 1 out]
        n267 = Equal?(x=w388, y=w390) -> (x = y?=w397:bool)
        n268 = Split Number(x=w391) -> (lo(x)=w389:u8)  [unwired: 1 out]
        n269 = Compound Arithmetic op=AND(w397, w382) -> (w384:bool)
        n270 = feedback #44(u8 0) -> (w394:u8)
        n271 = feedback-in #44(w389) -> ()
        n272 = feedback #45(FALSE) -> (w393:bool)
        n273 = feedback-in #45(w384) -> ()
        n274 = Select(t=w394, s=w393, f=u8 0) -> (s? t:f=w401:u8)
      }
      frame 255 {
        w403 = u32 536870912  # 2^29
        n275 = Not(x=w410) -> (.not. x?=w409:bool)
        n276 = feedback #46(FALSE) -> (w412:bool)
        n277 = Or(x=w412, y=w409) -> (x .or. y?=w413:bool)
        n278 = feedback #47(FALSE ("new data")) -> (w407:bool)
        n279 = Not(x=w407) -> (.not. x?=w411:bool)
        n280 = And(x=w413, y=w411) -> (x .and. y?=w406:bool)
        n281 = feedback-in #46(w406) -> ()
        n282 = call "_FPGA_MSProcess_DataReader.vi"("Read"=w406) -> ("Element"=w422:u64, "new data"=w408:bool)
        n283 = feedback-in #47(w408) -> ()
        n284 = xnode ("Register Write")("Data"=FALSE) -> ()  [unwired: 1 in, 1 out]
        n285 = Split Number(x=w422) -> (hi(x)=w418:u32, lo(x)=w420:u32)
        n286 = xnode ("Register Write")("Data"=w403) -> ()  [unwired: 1 in, 1 out]
        n287 = Equal?(x=w418, y=w420) -> (x = y?=w427:bool)
        n288 = Split Number(x=w418) -> (lo(x)=w421:u16)  [unwired: 1 out]
        n289 = Split Number(x=w421) -> (lo(x)=w419:u8)  [unwired: 1 out]
        n290 = Compound Arithmetic op=AND(w427, w408) -> (w415:bool)
        n291 = feedback #48(u8 0) -> (w424:u8)
        n292 = feedback-in #48(w419) -> ()
        n293 = feedback #49(FALSE) -> (w423:bool)
        n294 = feedback-in #49(w415) -> ()
        n295 = Select(t=w424, s=w423, f=w414) -> (s? t:f=w431:u8)
      }
      frame 1 {
        n296 = Equal To 0?(x=w440) -> (x = 0?=w439:bool)
        n297 = Compound Arithmetic op=AND(w434, w439) -> (w438:bool)
        n298 = feedback #50() -> (w436:bool)  [unwired: 1 in]
        n299 = call "_FPGA_MSProcess_ParameterHandler.vi"("Init"=w441, "Count Increse"=w436) -> ("Count"=w435:u8, "U64 Data"=w444:u64)
        n300 = feedback #51() -> (w451:u32)  [unwired: 1 in]
        n301 = feedback #52() -> (w452:u32)  [unwired: 1 in]
        n302 = feedback #53() -> (w455:u32)  [unwired: 1 in]
        n303 = feedback #54() -> (w432:bool)  [unwired: 1 in]
        n304 = case shown="3" w435 {
          tunnel: w444 -> [_ w470 w481 _ _]
          tunnel: [w463 w469 w479 w483 w505] -> w456
          tunnel: [w462 w468 w480 w484 w506] -> w454
          tunnel: [w461 _ w474 w485 w507] -> w453
          tunnel: w455 -> [w463 _ w479 w483 w505]
          tunnel: w452 -> [w462 _ w480 w484 w506]
          tunnel: w451 -> [w461 _ _ w485 w507]
          tunnel: [w460 w467 w478 w491 w504] -> w450
          tunnel: [w459 w466 w477 w489 w503] -> w449
          tunnel: [w458 w465 w476 w487 w502] -> w448
          tunnel: w447 -> [w460 w467 w478 w490 w504]
          tunnel: w446 -> [w459 w466 w477 w488 w503]
          tunnel: w445 -> [w458 w465 w476 w486 w502]
          tunnel: w443 -> [w457 w464 w475 w493 _]
          tunnel: [w457 w464 w475 w493 u8 255] -> w442
          tunnel: w438 -> [_ _ _ w492 _]
          tunnel: [_ _ _ w492 _] -> w437
          tunnel: [_ _ w471 w482 _] -> w433
          tunnel: w432 -> [_ _ _ w482 _]
          frame 0, Default {
          }
          frame 1 {
            n305 = Split Number(x=w470) -> (hi(x)=w469:u32, lo(x)=w468:u32)
          }
          frame 2 {
            n306 = Split Number(x=w481) -> (hi(x)=w473:u32, lo(x)=w474:u32)
            n307 = Split Number(x=w473) -> (lo(x)=w472:u16)  [unwired: 1 out]
            n308 = Not Equal To 0?(x=w472) -> (x != 0?=w471:bool)
          }
          frame 3 {
            n309 = case shown="True" w492 {
              tunnel: [w496 w500] -> w491
              tunnel: w490 -> [w496 _]
              tunnel: [w495 w499] -> w489
              tunnel: w488 -> [w495 _]
              tunnel: [w494 w498] -> w487
              tunnel: w486 -> [w494 _]
              tunnel: w483 -> [_ w500]
              tunnel: w484 -> [_ w499]
              tunnel: w485 -> [_ w498]
              tunnel: w482 -> [_ w497]
              frame False {
              }
              frame True {
                n310 = xnode ("Register Write")("Data"=w497) -> ()  [unwired: 1 in, 1 out]
              }
            }
          }
          frame 4 {
          }
        }
        n311 = feedback-in #50(w437) -> ()
        n312 = feedback-in #51(w453) -> ()
        n313 = feedback-in #52(w454) -> ()
        n314 = feedback-in #53(w456) -> ()
        n315 = feedback-in #54(w433) -> ()
      }
      frame 2 {
        n316 = call "_FPGA_MSProcess_ParameterHandler.vi"("Init"=w511) -> ("Count"=w508:u8, "U64 Data"=w512:u64)  [unwired: 1 in]
        n317 = case shown="0, Default" w508 {
          tunnel: w512 -> [_ _]
          tunnel: [w518 u32 0] -> w516
          tunnel: w515 -> [w518 _]
          tunnel: w514 -> [w517 _]
          tunnel: [w517 u8 255] -> w513
          frame 0, Default {
          }
          frame 1 {
          }
        }
      }
      frame 3 {
        n318 = feedback #55() -> (w523:bool)  [unwired: 1 in]
        n319 = call "_FPGA_MSProcess_ParameterHandler.vi"("Init"=w531, "Count Increse"=w523) -> ("Count"=w521:u8, "U64 Data"=w532:u64)
        n320 = feedback #56() -> (w526:bool)  [unwired: 1 in]
        n321 = case shown="0, Default" w521 {
          tunnel: w532 -> [_ w537 w544 _ _]
          tunnel: [_ _ TRUE _ _] -> w527
          tunnel: w526 -> [_ _ _ w545 _]
          tunnel: w525 -> [w533 w534 w538 w546 _]
          tunnel: [_ _ _ w547 _] -> w524
          tunnel: [w533 w534 w538 w546 u8 255] -> w522
          frame 0, Default {
          }
          frame 1 {
            n322 = Split Number(x=w537) -> (hi(x)=w536:u32, lo(x)=w535:u32)
            n323 = xnode ("Register Read")("Data"=w535) -> ()  [unwired: 1 in, 1 out]
            n324 = xnode ("Register Read")("Data"=w536) -> ()  [unwired: 1 in, 1 out]
          }
          frame 2 {
            n325 = Split Number(x=w544) -> (hi(x)=w541:u32, lo(x)=w540:u32)
            n326 = Split Number(x=w541) -> (lo(x)=w543:u16)  [unwired: 1 out]
            n327 = Split Number(x=w543) -> (lo(x)=w542:u8)  [unwired: 1 out]
            n328 = xnode ("Register Read")("Data"=w542) -> ()  [unwired: 1 in, 1 out]
            n329 = xnode ("Register Read")("Data"=w540) -> ()  [unwired: 1 in, 1 out]
          }
          frame 3 {
            n330 = case shown="True" w545 {
              frame False {
              }
              frame True {
                n331 = xnode ("FIFO Method Node")("Element"=TRUE, "Timeout"=0) -> ()  [unwired: 1 in, 2 out]
              }
            }
            n332 = xnode ("Register Read")("Data"=w545) -> ()  [unwired: 1 in, 1 out]
            n333 = xnode ("Register Write")() -> ("Data"=w548:bool)  [unwired: 1 in, 1 out]
            n334 = call <instrlib>:"Detect Falling Edge.vi"("signal"=w548) -> ("edge detected"=w547:bool)  [unwired: 14 in]
          }
          frame 4 {
          }
        }
        n335 = feedback-in #55(w524) -> ()
        n336 = feedback-in #56(w527) -> ()
      }
      frame 4 {
        n337 = feedback #57() -> (w553:bool)  [unwired: 1 in]
        n338 = call "_FPGA_MSProcess_ParameterHandler.vi"("Init"=w562, "Count Increse"=w553) -> ("Count"=w552:u8, "U64 Data"=w563:u64)
        n339 = feedback #58() -> (w558:bool)  [unwired: 1 in]
        n340 = case shown="1" w552 {
          tunnel: w563 -> [_ w568 w578 _ _]
          tunnel: [_ _ TRUE _ _] -> w557
          tunnel: w558 -> [_ _ _ w581 _]
          tunnel: w556 -> [w564 w565 w569 w580 _]
          tunnel: [w564 w565 w569 w580 u8 255] -> w555
          tunnel: [_ _ _ w579 _] -> w554
          frame 0, Default {
          }
          frame 1 {
            n341 = Split Number(x=w568) -> (hi(x)=w567:u32, lo(x)=w566:u32)
            n342 = xnode ("Register Read")("Data"=w567) -> ()  [unwired: 1 in, 1 out]
            n343 = xnode ("Register Read")("Data"=w566) -> ()  [unwired: 1 in, 1 out]
          }
          frame 2 {
            n344 = Split Number(x=w578) -> (hi(x)=w576:u32, lo(x)=w577:u32)
            n345 = Split Number(x=w576) -> (lo(x)=w575:u16)  [unwired: 1 out]
            n346 = Split Number(x=w575) -> (lo(x)=w574:u8)  [unwired: 1 out]
            n347 = Number To Boolean Array(number=w574) -> (Boolean array=w573:bool[])
            n348 = Index Array(array=w573, index=0) -> (element=w572:bool)
            n349 = xnode ("Register Read")("Data"=w577) -> ()  [unwired: 1 in, 1 out]
            n350 = xnode ("Register Read")("Data"=w572) -> ()  [unwired: 1 in, 1 out]
          }
          frame 3 {
            n351 = xnode ("Register Read")("Data"=w581) -> ()  [unwired: 1 in, 1 out]
            n352 = xnode ("Register Write")() -> ("Data"=w582:bool)  [unwired: 1 in, 1 out]
            n353 = call <instrlib>:"Detect Falling Edge.vi"("signal"=w582) -> ("edge detected"=w579:bool)  [unwired: 14 in]
          }
          frame 4 {
          }
        }
        n354 = feedback-in #57(w554) -> ()
        n355 = feedback-in #58(w557) -> ()
      }
      frame 5 {
        n356 = feedback #59(FALSE ("Not Conj?")) -> (w592:bool)
        n357 = call "_FPGA_MSProcess_ParameterHandler.vi"("Init"=w597, "Count Increse"=w592) -> ("Count"=w584:u8, "U64 Data"=w585:u64)
        n358 = feedback #60(cluster{"Ratio*2^15":u16, "CycleDiff":u64}[] [{"Ratio*2^15"=0, "CycleDiff"=0}, {"Ratio*2^15"=0, "CycleDiff"=0}, {"Ratio*2^15"=0, "CycleDiff"=0}, {"Ratio*2^15"=0, "CycleDiff"=0}, {"Ratio*2^15"=0, "CycleDiff"=0}, {"Ratio*2^15"=0, "CycleDiff"=0}, {"Ratio*2^15"=0, "CycleDiff"=0}, {"Ratio*2^15"=0, "CycleDiff"=0}, {"Ratio*2^15"=0, "CycleDiff"=0}, {"Ratio*2^15"=0, "CycleDiff"=0}, {"Ratio*2^15"=0, "CycleDiff"=0}, {"Ratio*2^15"=0, "CycleDiff"=0}, {"Ratio*2^15"=0, "CycleDiff"=0}, {"Ratio*2^15"=0, "CycleDiff"=0}, {"Ratio*2^15"=0, "CycleDiff"=0}, {"Ratio*2^15"=0, "CycleDiff"=0}] ("ConjArr")) -> (w601:cluster{"Ratio*2^15":u16, "CycleDiff":u64}[])
        n359 = feedback #61() -> (w603:u32)  [unwired: 1 in]
        n360 = feedback #62() -> (w604:u8)  [unwired: 1 in]
        n361 = case shown="2..17" w584 {
          selector: w584 -> [_ _ w619 _ _ _]
          tunnel: w585 -> [_ w617 w618 _ _ _]
          tunnel: [w608 w614 w635 w640 w646 w650] -> w598
          tunnel: [w607 w613 w634 w639 w645 w649] -> w599
          tunnel: w604 -> [w608 _ w635 w640 w646 w650]
          tunnel: w603 -> [w607 _ w634 w639 w645 w649]
          tunnel: w601 -> [w606 w612 w625 w638 w644 w648]
          tunnel: [w606 w612 w621 w638 w644 w648] -> w600
          tunnel: [_ _ _ w636 w642 _] -> w593
          tunnel: [_ _ _ w636 _ _] -> w591
          tunnel: w590 -> [w605 w611 w620 w637 w641 _]
          tunnel: [w605 w611 w620 w637 w641 u8 255] -> w589
          tunnel: w588 -> [_ _ _ w636 _ _]
          tunnel: w586 -> [_ _ _ _ w643 _]
          frame 0, Default {
          }
          frame 1 {
            n362 = Split Number(x=w617) -> (hi(x)=w616:u32, lo(x)=w613:u32)
            n363 = Split Number(x=w616) -> (lo(x)=w615:u16)  [unwired: 1 out]
            n364 = Split Number(x=w615) -> (hi(x)=w610:u8, lo(x)=w614:u8)
            n365 = Not Equal To 0?(x=w610) -> (x != 0?=w609:bool)
            n366 = xnode ("Register Write")("Data"=w609) -> ()  [unwired: 1 in, 1 out]
          }
          frame 2..17 {
            n367 = Split Number(x=w618) -> (hi(x)=w633:u32, lo(x)=w629:u32)
            n368 = Split Number(x=w633) -> (hi(x)=w626:u16, lo(x)=w632:u16)
            n369 = Subtract(x=w619, y=u8 2) -> (x-y=w622:u8)
            n370 = Join Numbers(hi=u16 0, lo=w632) -> ((hi.lo)=w630:u32)
            n371 = Join Numbers(hi=w630, lo=w629) -> ((hi.lo)=w627:u64)
            n372 = Bundle By Name(cluster=cluster{"Ratio*2^15":u16, "CycleDiff":u64} {"Ratio*2^15"=0, "CycleDiff"=0} ("Cluster"), "Ratio*2^15"=w626, "CycleDiff"=w627) -> (w624:cluster{"Ratio*2^15":u16, "CycleDiff":u64})
            n373 = Replace Array Subset(array=w625, new element=w624, index=w622) -> (w621:cluster{"Ratio*2^15":u16, "CycleDiff":u64}[])
          }
          frame 18 {
          }
          frame 19 {
            n374 = Not(x=w643) -> (.not. x?=w642:bool)
          }
          frame 20 {
          }
        }
        n375 = feedback-in #59(w593) -> ()
        n376 = feedback-in #60(w600) -> ()
        n377 = feedback-in #61(w599) -> ()
        n378 = feedback-in #62(w598) -> ()
      }
      frame 6 {
        n379 = call "_FPGA_MSProcess_ParameterHandler.vi"("Init"=w655) -> ("Count"=w651:u8, "U64 Data"=w658:u64)  [unwired: 1 in]
        n380 = case shown="1" w651 {
          tunnel: w658 -> [_ w675 _]
          tunnel: w657 -> [w659 w666 _]
          tunnel: [w659 w666 u8 255] -> w656
          frame 0, Default {
          }
          frame 1 {
            n381 = Split Number(x=w675) -> (hi(x)=w674:u32, lo(x)=w664:u32)
            n382 = Split Number(x=w674) -> (lo(x)=w673:u16)  [unwired: 1 out]
            n383 = Split Number(x=w673) -> (lo(x)=w672:u8)  [unwired: 1 out]
            n384 = Split Number(x=w664) -> (hi(x)=w662:u16, lo(x)=w663:u16)
            n385 = Number To Boolean Array(number=w672) -> (Boolean array=w671:bool[])
            n386 = Index Array(array=w671, index #1=2 ("index"), index #2=1 ("index"), index #3=0 ("index")) -> (element #1=w660:bool, element #2=w667:bool, element #3=w668:bool)
            n387 = xnode ("Register Write")("Data"=FALSE) -> ()  [unwired: 1 in, 1 out]
            n388 = xnode ("Register Write")("Data"=w660) -> ()  [unwired: 1 in, 1 out]
            n389 = xnode ("Register Read")("Data"=w667) -> ()  [unwired: 1 in, 1 out]
            n390 = xnode ("Register Write")("Data"=w668) -> ()  [unwired: 1 in, 1 out]
            n391 = xnode ("Register Write")("Data"=w662) -> ()  [unwired: 1 in, 1 out]
            n392 = xnode ("Register Read")("Data"=w663) -> ()  [unwired: 1 in, 1 out]
          }
          frame 2 {
          }
        }
      }
      frame 7 {
        n393 = feedback #63() -> (w677:bool)  [unwired: 1 in]
        n394 = call "_FPGA_MSProcess_ParameterHandler.vi"("Init"=w683, "Count Increse"=w677) -> ("Count"=w679:u8, "U64 Data"=w686:u64)
        n395 = case shown="0, Default" w679 {
          tunnel: w686 -> [_ w690 _ _ _]
          tunnel: w685 -> [w687 w689 w695 w696 _]
          tunnel: [w687 w689 w695 w696 u8 255] -> w684
          tunnel: [_ _ w691 w697 _] -> w678
          tunnel: w677 -> [_ _ _ _ _]
          frame 0, Default {
          }
          frame 1 {
            n396 = Split Number(x=w690) -> (lo(x)=w688:u32)  [unwired: 1 out]
            n397 = xnode ("Register Write")("Data"=w688) -> ()  [unwired: 1 in, 1 out]
          }
          frame 2 {
            n398 = xnode ("FIFO Method Node")("Element"=TRUE, "Timeout"=0) -> ("Timed Out?"=w692)  [unwired: 1 in, 1 out]
            n399 = Not(x=w692) -> (.not. x?=w691:bool)
          }
          frame 3 {
            n400 = xnode ("Register Write")() -> ("Data"=w698:bool)  [unwired: 1 in, 1 out]
            n401 = call <instrlib>:"Detect Falling Edge.vi"("signal"=w698) -> ("edge detected"=w697:bool)  [unwired: 14 in]
          }
          frame 4 {
          }
        }
        n402 = feedback-in #63(w678) -> ()
      }
      frame 8 {
        n403 = feedback #64() -> (w700:bool)  [unwired: 1 in]
        n404 = feedback #65() -> (w705:bool)  [unwired: 1 in]
        n405 = call "_FPGA_MSProcess_ParameterHandler.vi"("Init"=w714, "Count Increse"=w705) -> ("Count"=w704:u8, "U64 Data"=w717:u64)
        n406 = feedback #66() -> (w702:u32)  [unwired: 1 in]
        n407 = feedback #67() -> (w710:u32)  [unwired: 1 in]
        n408 = feedback #68() -> (w712:bool)  [unwired: 1 in]
        n409 = case shown="1" w704 {
          tunnel: w717 -> [_ w719 w729 _ _]
          tunnel: w716 -> [w718 w722 w731 w742 _]
          tunnel: [w718 w722 w731 w742 u8 255] -> w715
          tunnel: [_ TRUE TRUE _ _] -> w713
          tunnel: w712 -> [_ _ _ w746 _]
          tunnel: [_ w720 w728 w741 _] -> w711
          tunnel: w710 -> [_ _ w728 w741 _]
          tunnel: [_ _ _ w733 _] -> w706
          tunnel: [_ _ w724 w739 _] -> w703
          tunnel: w702 -> [_ _ _ w739 _]
          tunnel: [_ _ w723 w735 _] -> w701
          tunnel: w700 -> [_ _ _ w734 _]
          frame 0, Default {
          }
          frame 1 {
            n410 = Split Number(x=w719) -> (lo(x)=w720:u32)  [unwired: 1 out]
          }
          frame 2 {
            n411 = Split Number(x=w729) -> (lo(x)=w724:u32)  [unwired: 1 out]
            n412 = xnode ("Register Read")() -> ("Data"=w727:u8)  [unwired: 1 in, 1 out]
            n413 = Split Number(x=w724) -> (hi(x)=w726:u16)  [unwired: 1 out]
            n414 = Number To Boolean Array(number=w727) -> (Boolean array=w725:bool[])
            n415 = Index Array(array=w725, index=w726) -> (element=w723:bool)
          }
          frame 3 {
            n416 = xnode ("Register Read")() -> ("Data"=w740:u8)  [unwired: 1 in, 1 out]
            n417 = Split Number(x=w739) -> (hi(x)=w738:u16, lo(x)=w736:u16)
            n418 = Number To Boolean Array(number=w740) -> (Boolean array=w737:bool[])
            n419 = feedback #69() -> (w744:bool)  [unwired: 1 in]
            n420 = call-poly <instrlib>:"Count Down.vi"("count in"=w741, "load"=w746, "decrement"=w744) -> ("terminal count"=w743:bool)  [unwired: 11 in, 1 out]
            n421 = Index Array(array=w737, index=w738) -> (element=w735:bool)
            n422 = Not(x=w743) -> (.not. x?=w745:bool)
            n423 = feedback-in #69(w745) -> ()
            n424 = case shown="3" w736 {
              tunnel: w735 -> [_ w749 w752 w755]
              tunnel: w734 -> [_ w750 w753 w756]
              tunnel: [FALSE w748 w751 w754] -> w732
              frame 0, Default {
              }
              frame 1 {
                n425 = Compound Arithmetic op=AND(invert w749, w750) -> (w748:bool)
              }
              frame 2 {
                n426 = Compound Arithmetic op=AND(w752, invert w753) -> (w751:bool)
              }
              frame 3 {
                n427 = Not Equal?(x=w755, y=w756) -> (x != y?=w754:bool)
              }
            }
            n428 = Or(x=w743, y=w732) -> (x .or. y?=w733:bool)
          }
          frame 4 {
          }
        }
        n429 = feedback-in #64(w701) -> ()
        n430 = feedback-in #65(w706) -> ()
        n431 = feedback-in #66(w703) -> ()
        n432 = feedback-in #67(w711) -> ()
        n433 = feedback-in #68(w713) -> ()
      }
      frame 9 {
        n434 = call "_FPGA_MSProcess_ParameterHandler.vi"("Init"=w763) -> ("Count"=w764:u8, "U64 Data"=w765:u64)  [unwired: 1 in]
        n435 = case shown="2" w764 {
          tunnel: w765 -> [_ w770 _]
          tunnel: w759 -> [w766 w767 _]
          tunnel: [w766 w767 u8 255] -> w758
          frame 0, Default {
          }
          frame 1 {
            n436 = Split Number(x=w770) -> (hi(x)=w769:u32, lo(x)=w768:u32)
            n437 = xnode ("Register Read")("Data"=w769) -> ()  [unwired: 1 in, 1 out]
            n438 = xnode ("Register Read")("Data"=w768) -> ()  [unwired: 1 in, 1 out]
          }
          frame 2 {
          }
        }
      }
      frame 10 {
        n439 = call "_FPGA_MSProcess_ParameterHandler.vi"("Init"=w782) -> ("Count"=w783:u8, "U64 Data"=w773:u64)  [unwired: 1 in]
        n440 = Split Number(x=w773) -> (lo(x)=w774:u32)  [unwired: 1 out]
        n441 = Split Number(x=w774) -> (lo(x)=w775:u16)  [unwired: 1 out]
        n442 = Number To Boolean Array(number=w775) -> (Boolean array=w776:bool[])
        n443 = Boolean Array To Number(Boolean array=w776) -> (number=w772:fxp<+/-,16,14>)
        n444 = case shown="1" w783 {
          tunnel: w778 -> [w784 w786 w788 w790 _]
          tunnel: [w784 w786 w788 w790 u8 255] -> w777
          tunnel: w772 -> [_ w785 w787 w789 _]
          frame 0, Default {
          }
          frame 1 {
            n445 = xnode ("Register Write")("Data"=w785) -> ()  [unwired: 1 in, 1 out]
          }
          frame 2 {
            n446 = xnode ("Register Write")("Data"=w787) -> ()  [unwired: 1 in, 1 out]
          }
          frame 3 {
            n447 = xnode ("Register Write")("Data"=w789) -> ()  [unwired: 1 in, 1 out]
          }
          frame 4 {
          }
        }
      }
      frame 11 {
        n448 = call "_FPGA_MSProcess_ParameterHandler.vi"("Init"=w801) -> ("Count"=w802:u8, "U64 Data"=w793:u64)  [unwired: 1 in]
        n449 = Split Number(x=w793) -> (lo(x)=w794:u32)  [unwired: 1 out]
        n450 = Split Number(x=w794) -> (lo(x)=w795:u16)  [unwired: 1 out]
        n451 = Split Number(x=w795) -> (lo(x)=w792:u8)  [unwired: 1 out]
        n452 = case shown="0, Default" w802 {
          tunnel: w797 -> [w803 w805 w807 w809 _]
          tunnel: [w803 w805 w807 w809 u8 255] -> w796
          tunnel: w792 -> [_ w804 w806 w808 _]
          frame 0, Default {
          }
          frame 1 {
            n453 = xnode ("Register Write")("Data"=w804) -> ()  [unwired: 1 in, 1 out]
          }
          frame 2 {
            n454 = xnode ("Register Write")("Data"=w806) -> ()  [unwired: 1 in, 1 out]
          }
          frame 3 {
            n455 = xnode ("Register Write")("Data"=w808) -> ()  [unwired: 1 in, 1 out]
          }
          frame 4 {
          }
        }
      }
      frame 12 {
        n456 = feedback #70() -> (w811:bool)  [unwired: 1 in]
        n457 = call "_FPGA_MSProcess_ParameterHandler.vi"("Init"=w818, "Count Increse"=w811) -> ("Count"=w819:u8, "U64 Data"=w820:u64)
        n458 = case shown="1" w819 {
          tunnel: w820 -> [_ w823 _ _ _]
          tunnel: w814 -> [w821 w824 w827 w830 _]
          tunnel: [w821 w824 w827 w830 u8 255] -> w813
          tunnel: [_ _ TRUE TRUE _] -> w812
          frame 0, Default {
          }
          frame 1 {
            n459 = Split Number(x=w823) -> (lo(x)=w822:u32)  [unwired: 1 out]
            n460 = xnode ("Register Write")("Data"=w822) -> ()  [unwired: 1 in, 1 out]
          }
          frame 2 {
            n461 = xnode ("Register Write")("Data"=TRUE) -> ()  [unwired: 1 in, 1 out]
          }
          frame 3 {
            n462 = xnode ("Register Write")("Data"=FALSE) -> ()  [unwired: 1 in, 1 out]
          }
          frame 4 {
          }
        }
        n463 = feedback-in #70(w812) -> ()
      }
      frame 13 {
        n464 = call "_FPGA_MSProcess_ParameterHandler.vi"("Init"=w841) -> ("Count"=w842:u8, "U64 Data"=w835:u64)  [unwired: 1 in]
        n465 = Split Number(x=w835) -> (lo(x)=w832:u32)  [unwired: 1 out]
        n466 = Number To Boolean Array(number=w832) -> (Boolean array=w834:bool[])
        n467 = Boolean Array To Number(Boolean array=w834) -> (number=w833:fxp<+,32,32>)
        n468 = case shown="1" w842 {
          tunnel: w837 -> [w843 w845 w847 w849 _]
          tunnel: [w843 w845 w847 w849 u8 255] -> w836
          tunnel: w833 -> [_ w844 w846 w848 _]
          frame 0, Default {
          }
          frame 1 {
            n469 = xnode ("Register Write")("Data"=w844) -> ()  [unwired: 1 in, 1 out]
          }
          frame 2 {
            n470 = xnode ("Register Write")("Data"=w846) -> ()  [unwired: 1 in, 1 out]
          }
          frame 3 {
            n471 = xnode ("Register Write")("Data"=w848) -> ()  [unwired: 1 in, 1 out]
          }
          frame 4 {
          }
        }
      }
      frame 20 {
        n472 = feedback #71() -> (w857:bool)  [unwired: 1 in]
        n473 = Or(x=w857, y=w852) -> (x .or. y?=w859:bool)
        n474 = call "_FPGA_MSProcess_DataReader.vi"("Read"=w859) -> ("Element"=w853:u64, "new data"=w851:bool)
        n475 = Not Equal?(x=u64 18446744073709551615 ("y"), y=w853) -> (x != y?=w854:bool)
        n476 = feedback-in #71(w854) -> ()
        n477 = case shown="True" w851 {
          tunnel: w856 -> [w864 w871]
          tunnel: w853 -> [w866 _]
          tunnel: [w863 w871] -> w855
          tunnel: w854 -> [w865 _]
          frame True {
            n478 = case shown="True" w865 {
              tunnel: w866 -> [_ w869]
              tunnel: w864 -> [_ w868]
              tunnel: [u8 255 ("f") w868] -> w863
              frame False {
              }
              frame True {
                n479 = xnode ("FIFO Method Node")("Element"=w869, "Timeout"=0) -> ()  [unwired: 1 in, 2 out]
              }
            }
          }
          frame False {
          }
        }
      }
      frame 21 {
        # "Aux start conj index"
        # "Active"
        n480 = Equal To 0?(x=w876) -> (x = 0?=w875:bool)
        n481 = feedback #72() -> (w888:u8)  [unwired: 1 in]
        n482 = feedback #73() -> (w883:u64)  [unwired: 1 in]
        n483 = feedback #74() -> (w877:u32)  [unwired: 1 in]
        n484 = feedback #75() -> (w874:bool)  [unwired: 1 in]
        n485 = Compound Arithmetic op=AND(w874, w872, w875) -> (w873:bool)
        n486 = call "_FPGA_MSProcess_ParameterHandler.vi"("Init"=w890, "Count Increse"=w873) -> ("Count"=w893:u8, "U64 Data"=w894:u64)
        n487 = case shown="9" w893 {
          tunnel: w894 -> [_ w899 w906 w908 _ w917 w924 w929 w936 _ _]
          tunnel: w892 -> [w897 w898 w901 w909 w911 w915 w920 w927 w932 w937 w961]
          tunnel: [w897 w898 w901 w909 w911 w915 w920 w927 w932 w937 w960] -> w891
          tunnel: [_ _ _ _ _ _ _ _ _ TRUE _] -> w889
          tunnel: w874 -> [_ _ _ _ _ _ _ _ _ _ _]
          tunnel: [w895 _ w900 w907 w910 w913 w918 w925 w930 w938 w957] -> w887
          tunnel: w888 -> [w895 _ _ w907 w910 w913 w918 w925 w930 w938 w957]
          tunnel: w872 -> [_ _ _ _ _ _ _ _ _ _ w947]
          tunnel: [_ _ _ _ _ _ _ _ _ _ w952] -> w886
          tunnel: w885 -> [_ _ _ _ _ _ _ _ _ _ w962]
          tunnel: [w896 _ _ w908 w912 w914 w919 w926 w931 w939 w963] -> w884
          tunnel: w883 -> [w896 _ _ _ w912 w914 w919 w926 w931 w939 w963]
          tunnel: [_ _ _ _ _ _ _ _ _ _ TRUE ("out")] -> w882
          tunnel: [_ _ _ _ _ w916 _ w928 _ w940 w949] -> w878
          tunnel: w877 -> [_ _ _ _ _ _ w922 _ w934 w940 w949]
          frame 0, Default {
          }
          frame 1 {
            n488 = xnode ("Register Write")("Data"=w899) -> ()  [unwired: 1 in, 1 out]
          }
          frame 2 {
            n489 = Split Number(x=w906) -> (hi(x)=w904:u32, lo(x)=w905:u32)
            n490 = Split Number(x=w904) -> (lo(x)=w903:u16)  [unwired: 1 out]
            n491 = Split Number(x=w903) -> (hi(x)=w902:u8, lo(x)=w900:u8)
            n492 = xnode ("Register Write")("Data"=w902) -> ()  [unwired: 1 in, 1 out]
            n493 = xnode ("Register Write")("Data"=w905) -> ()  [unwired: 1 in, 1 out]
          }
          frame 3 {
          }
          frame 4 {
          }
          frame 5 {
            n494 = Split Number(x=w917) -> (lo(x)=w916:u32)  [unwired: 1 out]
          }
          frame 6 {
            n495 = Split Number(x=w924) -> (lo(x)=w923:u32)  [unwired: 1 out]
            n496 = Join Numbers(hi=w922, lo=w923) -> ((hi.lo)=w921:u64)
            n497 = xnode ("Register Write")("Data"=w921) -> ()  [unwired: 1 in, 1 out]
          }
          frame 7 {
            n498 = Split Number(x=w929) -> (lo(x)=w928:u32)  [unwired: 1 out]
          }
          frame 8 {
            n499 = Split Number(x=w936) -> (lo(x)=w935:u32)  [unwired: 1 out]
            n500 = Join Numbers(hi=w934, lo=w935) -> ((hi.lo)=w933:u64)
            n501 = xnode ("Register Write")("Data"=w933) -> ()  [unwired: 1 in, 1 out]
          }
          frame 9 {
          }
          frame 10 {
            n502 = Greater?(x=w963, y=w962) -> (0:w956:bool)
            n503 = feedback #76() -> (w945:u64)  [unwired: 1 in]
            n504 = call "_FPGA_StepwiseScan_DataReader.vi"("Read data"=w947, "Data in"=w945) -> ("End?"=w942:bool, "Valid?"=w943:bool, "Data out"=w946:u64)  [unwired: 6 in, 1 out]
            n505 = feedback-in #76(w946) -> ()
            n506 = call-poly <instrlib>:"Count Up.vi"("increment"=w947, "reset"=w943) -> ("count out"=w958:u8)  [unwired: 13 in]
            n507 = Greater Or Equal?(x=w958, y=w957) -> (x >= y?=w951:bool)
            n508 = call "_FPGA_Aux_Reg_Scale&Amp.vi"("Data in"=w946) -> ()
            n509 = feedback #77() -> (w955:bool)  [unwired: 1 in]
            n510 = Or(x=w951, y=w955) -> (x .or. y?=w944:bool)
            n511 = Not(x=w955) -> (.not. x?=w954:bool)
            n512 = Compound Arithmetic op=AND(invert w943, invert w942, w944) -> (w950:bool)
            n513 = feedback-in #77(w950) -> ()
            n514 = Compound Arithmetic op=AND(w950, w951, w956) -> (w953:bool)
            n515 = xnode ("Register Write")("Data"=w953) -> ()  [unwired: 1 in, 1 out]
            n516 = Select(t=u8 255, s=w942, f=w961) -> (s? t:f=w960:u8)
            n517 = And(x=w950, y=w954) -> (x .and. y?=w952:bool)
          }
        }
        n518 = feedback-in #72(w887) -> ()
        n519 = feedback-in #73(w884) -> ()
        n520 = feedback-in #74(w878) -> ()
        n521 = feedback-in #75(w889) -> ()
      }
      frame 22 {
        # "AuxDecyc, AuxAmp"
        # "TotalAuxCycle"
        n522 = Equal To 0?(x=w968) -> (x = 0?=w967:bool)
        n523 = feedback #78() -> (w970:u64)  [unwired: 1 in]
        n524 = feedback #79() -> (w966:bool)  [unwired: 1 in]
        n525 = Compound Arithmetic op=AND(w966, w964, w967) -> (w965:bool)
        n526 = call "_FPGA_MSProcess_ParameterHandler.vi"("Init"=w975, "Count Increse"=w965) -> ("Count"=w978:u8, "U64 Data"=w979:u64)
        n527 = case shown="10" w978 {
          tunnel: w979 -> [_ w990 w999 w1004 w1012 w1019 w1029 w1033 w1038 _ _]
          tunnel: [w989 w994 w1003 w1008 w1017 w1022 w1032 w1037 w1043 w1048 w1068] -> w985
          tunnel: [w988 w993 w1002 w1007 w1016 w1021 w1031 w1036 w1042 w1047 w1064] -> w984
          tunnel: [w987 w992 w1001 w1006 w1015 w1020 w1030 w1035 w1041 w1046 w1063] -> w983
          tunnel: w982 -> [w989 w994 w1003 w1008 w1017 w1022 w1032 w1037 w1043 w1048 w1061]
          tunnel: w981 -> [w988 w993 w1002 w1007 w1016 w1021 w1031 w1036 w1042 w1047 w1062]
          tunnel: w980 -> [w987 w992 w1001 w1006 w1015 w1020 w1030 w1035 w1041 w1046 w1063]
          tunnel: w977 -> [w986 w991 w1000 w1005 w1014 w1018 w1023 w1034 w1039 w1044 w1074]
          tunnel: [w986 w991 w1000 w1005 w1014 w1018 w1023 w1034 w1039 w1044 w1073] -> w976
          tunnel: [_ _ _ _ _ _ _ _ _ TRUE _] -> w974
          tunnel: w966 -> [_ _ _ _ _ _ _ _ _ _ _]
          tunnel: [_ _ _ _ _ _ _ _ _ _ w1056] -> w973
          tunnel: w972 -> [_ _ _ _ _ _ _ _ _ _ w1069]
          tunnel: [_ w990 _ w1004 _ _ _ w1033 w1040 w1045 w1075] -> w971
          tunnel: w970 -> [_ _ w996 _ w1010 _ _ _ w1040 w1045 w1075]
          tunnel: [_ _ _ _ _ _ _ _ _ _ TRUE] -> w969
          tunnel: w964 -> [_ _ _ _ _ _ _ _ _ _ w1052]
          frame 0, Default {
          }
          frame 1 {
          }
          frame 2 {
            n528 = Split Number(x=w996) -> (lo(x)=w995:u32)  [unwired: 1 out]
            n529 = Split Number(x=w999) -> (lo(x)=w998:u32)  [unwired: 1 out]
            n530 = Join Numbers(hi=w995, lo=w998) -> ((hi.lo)=w997:u64)
            n531 = xnode ("Register Write")("Data"=w997) -> ()  [unwired: 1 in, 1 out]
          }
          frame 3 {
          }
          frame 4 {
            n532 = Split Number(x=w1010) -> (lo(x)=w1009:u32)  [unwired: 1 out]
            n533 = Split Number(x=w1012) -> (lo(x)=w1011:u32)  [unwired: 1 out]
            n534 = Join Numbers(hi=w1009, lo=w1011) -> ((hi.lo)=w1013:u64)
            n535 = xnode ("Register Write")("Data"=w1013) -> ()  [unwired: 1 in, 1 out]
          }
          frame 5 {
            n536 = xnode ("Register Write")("Data"=w1019) -> ()  [unwired: 1 in, 1 out]
          }
          frame 6 {
            n537 = Split Number(x=w1029) -> (hi(x)=w1027:u32, lo(x)=w1028:u32)
            n538 = Split Number(x=w1027) -> (lo(x)=w1026:u16)  [unwired: 1 out]
            n539 = Split Number(x=w1026) -> (hi(x)=w1025:u8, lo(x)=w1024:u8)
            n540 = xnode ("Register Write")("Data"=w1025) -> ()  [unwired: 1 in, 1 out]
            n541 = xnode ("Register Write")("Data"=w1024) -> ()  [unwired: 1 in, 1 out]
            n542 = xnode ("Register Write")("Data"=w1028) -> ()  [unwired: 1 in, 1 out]
          }
          frame 7 {
          }
          frame 8 {
            n543 = call "_FPGA_Aux_Reg_Scale&Amp.vi"("Data in"=w1038) -> ()
          }
          frame 9 {
          }
          frame 10 {
            n544 = Join Numbers(hi=w1061, lo=w1062) -> ((hi.lo)=w1070:u64)
            n545 = xnode ("Register Read")() -> ("Data"=w1066:u8)  [unwired: 1 in, 1 out]
            n546 = Greater?(x=w1075, y=w1069) -> (0:w1065:bool)
            n547 = call "_FPGA_StepwiseScan_DataReader.vi"("Read data"=w1052, "Data in"=w1070) -> ("End?"=w1050:bool, "Valid?"=w1051:bool, "Data out"=w1071:u64)  [unwired: 6 in, 1 out]
            n548 = Split Number(x=w1071) -> (hi(x)=w1068:u32, lo(x)=w1064:u32)
            n549 = call-poly <instrlib>:"Count Up.vi"("increment"=w1052, "reset"=w1051) -> ("count out"=w1067:u8)  [unwired: 13 in]
            n550 = Greater Or Equal?(x=w1067, y=w1066) -> (x >= y?=w1054:bool)
            n551 = feedback #80() -> (w1058:bool)  [unwired: 1 in]
            n552 = Or(x=w1054, y=w1058) -> (x .or. y?=w1060:bool)
            n553 = Not(x=w1058) -> (.not. x?=w1057:bool)
            n554 = Compound Arithmetic op=AND(invert w1051, invert w1050, w1060) -> (w1055:bool)
            n555 = feedback-in #80(w1055) -> ()
            n556 = Compound Arithmetic op=AND(w1055, w1065, w1054) -> (w1059:bool)
            n557 = And(x=w1055, y=w1057) -> (x .and. y?=w1056:bool)
            n558 = xnode ("Register Write")("Data"=w1059) -> ()  [unwired: 1 in, 1 out]
            n559 = Select(t=u8 255, s=w1050, f=w1074) -> (s? t:f=w1073:u8)
          }
        }
        n560 = feedback-in #78(w971) -> ()
        n561 = feedback-in #79(w974) -> ()
      }
      frame 23 {
        # "Aux Forward/Backward"
        # "RF Forward/Backward"
        # "Continous scan"
        # "Aux Amp Incr * 2^71 upper"
        # "RF Amp Incr * 2^71 upper"
        # "Aux Amp Incr * 2^71 lower 32bits"
        # "RF Amp Incr * 2^71 lower 32bits"
        # "Amp Ini"
        # "Amp Final"
        n562 = Number To Boolean Array(number=w1081) -> (Boolean array=w1080:bool[])
        n563 = Index Array(array=w1080, index=0) -> (element=w1078:bool)
        n564 = And(x=w1086, y=w1078) -> (x .and. y?=w1085:bool)
        n565 = feedback #81() -> (w1094:u64)  [unwired: 1 in]
        n566 = feedback #82() -> (w1093:u64)  [unwired: 1 in]
        n567 = feedback #83() -> (w1097:u64)  [unwired: 1 in]
        n568 = feedback #84() -> (w1092:u64)  [unwired: 1 in]
        n569 = feedback #85() -> (w1083:u64)  [unwired: 1 in]
        n570 = feedback #86() -> (w1101:u64)  [unwired: 1 in]
        n571 = feedback #87() -> (w1096:bool)  [unwired: 1 in]
        n572 = call "_FPGA_MSProcess_ParameterHandler.vi"("Init"=w1109, "Count Increse"=w1096) -> ("Count"=w1112:u8, "U64 Data"=w1113:u64)
        n573 = feedback #88() -> (w1087:bool)  [unwired: 1 in]
        n574 = feedback #89() -> (w1082:bool)  [unwired: 1 in]
        n575 = feedback #90() -> (w1077:bool)  [unwired: 1 in]
        n576 = case shown="16" w1112 {
          tunnel: w1113 -> [_ w1119 w1126 w1129 w1135 w1140 w1147 w1156 w1161 w1167 w1172 w1181 w1189 w1199 w1212 _ _]
          tunnel: [w1117 w1121 w1128 w1131 w1138 w1141 w1148 w1157 w1162 w1169 w1177 w1186 w1196 w1207 w1220 w1235 w1250] -> w1115
          tunnel: w1114 -> [w1117 w1121 w1128 w1131 w1138 w1141 w1148 w1157 w1162 w1169 w1177 w1186 w1196 w1207 w1220 w1235 _]
          tunnel: w1111 -> [w1116 w1120 w1127 w1130 w1137 w1139 w1142 w1155 w1163 w1170 w1178 w1187 w1197 w1208 w1221 w1236 w1249]
          tunnel: [w1116 w1120 w1127 w1130 w1137 w1139 w1142 w1155 w1163 w1170 w1178 w1187 w1197 w1208 w1221 w1236 w1248] -> w1110
          tunnel: w1108 -> [_ _ _ _ _ _ _ _ _ _ _ _ _ _ _ _ _]
          tunnel: [_ _ _ _ _ _ _ _ _ _ _ _ _ _ _ _ TRUE] -> w1107
          tunnel: [_ _ _ _ _ _ _ _ _ _ _ _ _ _ _ _ w1260] -> w1104
          tunnel: [_ _ _ _ _ _ _ _ _ _ _ _ _ _ _ w1228 _] -> w1103
          tunnel: [_ w1119 _ w1129 _ _ _ _ w1161 w1168 w1176 w1185 w1195 w1206 w1219 w1232 w1288] -> w1102
          tunnel: w1101 -> [_ _ w1123 _ w1133 _ _ _ _ w1168 w1176 w1185 w1195 w1206 w1219 w1232 w1288]
          tunnel: [_ _ _ _ _ _ _ _ _ w1167 w1175 w1184 w1194 w1205 w1218 w1231 w1287] -> w1100
          tunnel: w1083 -> [_ _ _ _ _ _ _ _ _ _ w1175 w1184 w1194 w1205 w1218 w1231 w1287]
          tunnel: [_ _ _ _ _ _ _ _ _ _ w1172 w1180 w1190 w1204 w1217 w1234 w1284] -> w1099
          tunnel: [_ _ _ _ _ _ _ _ _ _ _ _ w1189 w1203 w1215 w1233 w1282] -> w1098
          tunnel: w1097 -> [_ _ _ _ _ _ _ _ _ _ _ w1180 w1190 w1204 w1217 w1234 w1284]
          tunnel: w1094 -> [_ _ _ _ _ _ _ _ _ _ _ _ _ w1203 w1215 w1233 w1282]
          tunnel: w1096 -> [_ _ _ _ _ _ _ _ _ _ _ _ _ _ _ _ w1260]
          tunnel: [_ _ _ _ _ _ _ _ _ _ _ _ _ w1199 w1216 w1225 w1283] -> w1095
          tunnel: w1093 -> [_ _ _ _ _ _ _ _ _ _ _ _ _ _ w1216 w1225 w1283]
          tunnel: w1092 -> [_ _ _ _ _ _ _ _ _ _ _ _ w1191 w1200 w1213 w1226 w1285]
          tunnel: [_ _ _ _ _ _ _ _ _ _ _ w1181 w1191 w1200 w1213 w1226 w1285] -> w1091
          tunnel: w1090 -> [_ _ _ _ _ _ _ _ _ _ _ _ _ _ _ w1230 _]
          tunnel: [_ _ _ _ _ _ _ w1150 w1160 w1166 w1174 w1183 w1193 w1202 w1214 w1227 w1255] -> w1089
          tunnel: w1082 -> [_ _ _ _ _ _ _ _ w1160 w1166 w1174 w1183 w1193 w1202 w1214 w1227 w1255]
          tunnel: [_ _ _ _ _ _ _ w1151 w1159 w1165 w1173 w1182 w1192 w1201 w1210 w1224 w1259] -> w1088
          tunnel: w1087 -> [_ _ _ _ _ _ _ _ w1159 w1165 w1173 w1182 w1192 w1201 w1210 w1224 w1259]
          tunnel: w1085 -> [_ _ _ _ _ _ _ _ _ _ _ _ _ _ _ _ w1261]
          tunnel: w1084 -> [_ _ _ _ _ _ _ _ _ _ _ _ _ _ _ w1223 _]
          tunnel: w1077 -> [_ _ _ _ _ _ _ _ w1158 w1164 w1171 w1179 w1188 w1198 w1209 w1222 w1243]
          tunnel: [_ _ _ _ _ _ _ w1149 w1158 w1164 w1171 w1179 w1188 w1198 w1209 w1222 w1243] -> w1076
          frame 0, Default {
          }
          frame 1 {
            n577 = xnode ("Register Write")("Data"=FALSE) -> ()  [unwired: 1 in, 1 out]
          }
          frame 2 {
            n578 = Split Number(x=w1123) -> (lo(x)=w1122:u32)  [unwired: 1 out]
            n579 = Split Number(x=w1126) -> (lo(x)=w1125:u32)  [unwired: 1 out]
            n580 = Join Numbers(hi=w1122, lo=w1125) -> ((hi.lo)=w1124:u64)
            n581 = xnode ("Register Write")("Data"=w1124) -> ()  [unwired: 1 in, 1 out]
          }
          frame 3 {
          }
          frame 4 {
            n582 = Split Number(x=w1133) -> (lo(x)=w1132:u32)  [unwired: 1 out]
            n583 = Split Number(x=w1135) -> (lo(x)=w1134:u32)  [unwired: 1 out]
            n584 = Join Numbers(hi=w1132, lo=w1134) -> ((hi.lo)=w1136:u64)
            n585 = xnode ("Register Write")("Data"=w1136) -> ()  [unwired: 1 in, 1 out]
          }
          frame 5 {
            n586 = xnode ("Register Write")("Data"=w1140) -> ()  [unwired: 1 in, 1 out]
          }
          frame 6 {
            n587 = Split Number(x=w1147) -> (hi(x)=w1145:u32, lo(x)=w1146:u32)
            n588 = Split Number(x=w1145) -> (lo(x)=w1144:u16)  [unwired: 1 out]
            n589 = Split Number(x=w1144) -> (hi(x)=w1143:u8)  [unwired: 1 out]
            n590 = xnode ("Register Write")("Data"=w1143) -> ()  [unwired: 1 in, 1 out]
            n591 = xnode ("Register Write")("Data"=w1146) -> ()  [unwired: 1 in, 1 out]
          }
          frame 7 {
            (unwired) 0 ("index")
            # "Continuous"
            # "forward, backward"
            # "AuxScale"
            n592 = Split Number(x=w1156) -> (hi(x)=w1152:u32, lo(x)=w1154:u32)
            n593 = Number To Boolean Array(number=w1154) -> (Boolean array=w1153:bool[])
            n594 = xnode ("Register Write")("Data"=w1152) -> ()  [unwired: 1 in, 1 out]
            n595 = Index Array(array=w1153) -> (element #1=w1149:bool, element #2=w1150:bool, element #3=w1151:bool)  [unwired: 3 in]
          }
          frame 8 {
            # "Amp Final"
          }
          frame 9 {
            # "Amp Initial"
          }
          frame 10 {
            # "RF Amp Increment * 2^71 lower"
          }
          frame 11 {
            # "RF Amp Increment * 2^71 upper"
          }
          frame 12 {
            # "Aux Amp Increment * 2^71 lower"
          }
          frame 13 {
            # "Aux Amp Increment * 2^71 upper"
          }
          frame 14 {
            # "Aux Bases"
            n596 = Split Number(x=w1212) -> (lo(x)=w1211:u32)  [unwired: 1 out]
            n597 = xnode ("Register Write")("Data"=w1211) -> ()  [unwired: 1 in, 1 out]
          }
          frame 15 {
            n598 = Equal To 0?(x=w1230) -> (x = 0?=w1229:bool)
            n599 = And(x=w1223, y=w1229) -> (x .and. y?=w1228:bool)
          }
          frame 16 {
            n600 = Compound Arithmetic op=OR(w1259, w1260, w1261) -> (w1242:bool)
            n601 = feedback #91() -> (w1265:u32)  [unwired: 1 in]
            n602 = Select(t=u32 0 ("index"), s=w1260, f=w1265) -> (s? t:f=w1263:u32)
            n603 = To Unsigned Quad Integer(1:w1263) -> (0:w1264:u64)
            n604 = Increment(x=w1263) -> (x+1=w1262:u32)
            n605 = feedback-in #91(w1262) -> ()
            n606 = Multiply(x=w1285, y=w1264) -> (x*y=w1280:u64)
            n607 = Multiply(x=w1284, y=w1264) -> (x*y=w1278:u64)
            n608 = Multiply(x=w1283, y=w1264) -> (x*y=w1269:u64)
            n609 = Multiply(x=w1282, y=w1264) -> (x*y=w1268:u64)
            n610 = Logical Shift(y=i16 -32 ("n"), x=w1278) -> (x << y=w1277:u64)
            n611 = Logical Shift(y=i16 -32 ("n"), x=w1268) -> (x << y=w1271:u64)
            n612 = xnode ("Register Write")("Data"=TRUE) -> ()  [unwired: 1 in, 1 out]
            n613 = Add(x=w1280, y=w1277) -> (x+y=w1275:u64)
            n614 = Add(x=w1269, y=w1271) -> (x+y=w1273:u64)
            n615 = Logical Shift(y=i16 -10 ("n"), x=w1275) -> (x << y=w1274:u64)
            n616 = Logical Shift(y=i16 -10 ("n"), x=w1273) -> (x << y=w1267:u64)
            n617 = Split Number(x=w1288) -> (hi(x)=w1245:u32, lo(x)=w1237:u32)
            n618 = Split Number(x=w1287) -> (hi(x)=w1244:u32, lo(x)=w1257:u32)
            n619 = To Unsigned Long Integer(number=w1274) -> (unsigned 32bit integer=w1258:u32)
            n620 = To Unsigned Long Integer(number=w1267) -> (unsigned 32bit integer=w1256:u32)
            n621 = Add(x=w1244, y=w1258) -> (x+y=w1252:u32)
            n622 = Subtract(x=w1244, y=w1258) -> (x-y=w1251:u32)
            n623 = Add(x=w1257, y=w1256) -> (x+y=w1239:u32)
            n624 = Subtract(x=w1257, y=w1256) -> (x-y=w1238:u32)
            n625 = Less Or Equal?(x=w1245, y=w1252) -> (x <= y?=w1246:bool)
            n626 = Greater Or Equal?(x=w1245, y=w1251) -> (x >= y?=w1247:bool)
            n627 = Build Array(w1246, w1247, w1255, w1243, w1242) -> (w1254:bool[])
            n628 = Boolean Array To Number(Boolean array=w1254) -> (number=w1253:u8)
            n629 = feedback #92() -> (w1241:u32)  [unwired: 1 in]
            n630 = feedback #93() -> (w1289:u32)  [unwired: 1 in]
            n631 = case shown="24, 25" w1253 {
              tunnel: w1252 -> [_ _ _ w1300 w1303 _]
              tunnel: w1251 -> [_ w1293 _ _ _ w1306]
              tunnel: [w1292 w1293 w1298 w1300 w1303 w1306] -> w1250
              tunnel: w1289 -> [w1292 _ _ _ _ _]
              tunnel: w1245 -> [_ _ w1298 _ _ _]
              tunnel: w1249 -> [w1291 w1295 _ w1301 w1304 w1307]
              tunnel: [w1291 w1295 u8 255 w1301 w1304 w1307] -> w1248
              tunnel: w1241 -> [w1290 _ _ _ _ _]
              tunnel: [w1290 w1294 w1297 w1299 w1302 w1305] -> w1240
              tunnel: w1239 -> [_ _ _ _ w1302 w1305]
              tunnel: w1238 -> [_ w1294 _ w1299 _ _]
              tunnel: w1237 -> [_ _ w1297 _ _ _]
              frame Default {
              }
              frame 16, 17 {
              }
              frame 18, 19, 21, 23, 26, 27, 29, 31 {
              }
              frame 20, 22 {
              }
              frame 28, 30 {
              }
              frame 24, 25 {
              }
            }
            n632 = xnode ("Register Write")("Data"=w1240) -> ()  [unwired: 1 in, 1 out]
            n633 = feedback-in #92(w1240) -> ()
            n634 = feedback-in #93(w1250) -> ()
          }
        }
        n635 = feedback-in #81(w1098) -> ()
        n636 = feedback-in #82(w1095) -> ()
        n637 = feedback-in #83(w1099) -> ()
        n638 = feedback-in #84(w1091) -> ()
        n639 = feedback-in #85(w1100) -> ()
        n640 = feedback-in #86(w1102) -> ()
        n641 = feedback-in #87(w1103) -> ()
        n642 = feedback-in #88(w1088) -> ()
        n643 = feedback-in #89(w1089) -> ()
        n644 = feedback-in #90(w1076) -> ()
      }
      frame 24 {
        # "Direction"
        # "Current Decyc"
        # "Target Decyc, Target 1/Decyc"
        # "Decyc Increment"
        n645 = Equal To 0?(x=w1318) -> (x = 0?=w1317:bool)
        n646 = Compound Arithmetic op=AND(w1316, w1317) -> (w1311:bool)
        n647 = feedback #94() -> (w1323:u64)  [unwired: 1 in]
        n648 = feedback #95() -> (w1319:u64)  [unwired: 1 in]
        n649 = feedback #96() -> (w1314:u64)  [unwired: 1 in]
        n650 = feedback #97() -> (w1312:bool)  [unwired: 1 in]
        n651 = call "_FPGA_MSProcess_ParameterHandler.vi"("Init"=w1325, "Count Increse"=w1312) -> ("Count"=w1328:u8, "U64 Data"=w1329:u64)
        n652 = feedback #98() -> (w1309:bool)  [unwired: 1 in]
        n653 = case shown="4" w1328 {
          tunnel: w1329 -> [_ w1339 w1346 w1353 _ _ _]
          tunnel: [w1338 w1343 w1345 w1355 w1366 w1377 w1386] -> w1315
          tunnel: [w1337 w1342 w1351 w1356 w1365 w1382 w1385] -> w1334
          tunnel: [w1336 w1341 w1350 w1357 w1364 w1383 w1389] -> w1333
          tunnel: w1332 -> [w1338 w1343 w1345 w1355 w1366 _ _]
          tunnel: w1331 -> [w1337 w1342 w1351 w1356 w1365 w1382 _]
          tunnel: w1330 -> [w1336 w1341 w1350 w1357 w1364 w1383 w1389]
          tunnel: w1327 -> [w1335 w1340 w1349 w1354 w1363 w1376 _]
          tunnel: [w1335 w1340 w1349 w1354 w1363 w1376 u8 255] -> w1326
          tunnel: [_ _ _ _ w1370 w1384 _] -> w1324
          tunnel: [_ _ w1346 w1361 w1367 w1379 _] -> w1322
          tunnel: w1323 -> [_ _ _ w1361 w1367 w1379 _]
          tunnel: w1321 -> [_ _ _ _ _ _ _]
          tunnel: [_ _ w1347 w1359 w1368 w1378 _] -> w1320
          tunnel: w1319 -> [_ _ _ w1359 w1368 w1380 _]
          tunnel: w1314 -> [_ _ w1348 w1360 w1369 w1374 w1387]
          tunnel: [_ w1339 w1348 w1360 w1369 w1374 _] -> w1313
          tunnel: w1311 -> [_ _ _ _ w1370 _ _]
          tunnel: [_ _ _ w1358 w1362 w1381 _] -> w1310
          tunnel: w1309 -> [_ _ _ _ w1362 w1381 _]
          tunnel: [_ _ _ _ _ TRUE _] -> w1308
          frame 0, Default {
          }
          frame 1 {
            # "Target Freq"
          }
          frame 2 {
            # "The Decycle increment may be very very small."
            # "Decyc increment"
            n654 = Join Numbers(hi=w1345, lo=u32 0) -> ((hi.lo)=w1347:u64)
          }
          frame 3 {
            n655 = Split Number(x=w1353) -> (lo(x)=w1352:u32)  [unwired: 1 out]
            n656 = xnode ("Register Read")("Data"=w1352) -> ()  [unwired: 1 in, 1 out]
            n657 = Greater?(x=w1360, y=w1359) -> (0:w1358:bool)
          }
          frame 4 {
          }
          frame 5 {
            n658 = Split Number(x=w1374) -> (hi(x)=w1373:u32)  [unwired: 1 out]
            n659 = Join Numbers(hi=w1373, lo=u32 0) -> ((hi.lo)=w1371:u64)
            n660 = call "_FPGA_DeCycAdder.vi"("DecycIncrement"=w1379, "CurrentDecyc in"=w1380, "TargetDecyc"=w1371, "Direction"=w1381) -> ("ReachTarget"=w1384:bool, "CurrentDecyc out"=w1378:u64)  [unwired: 6 in]
            n661 = Split Number(x=w1378) -> (hi(x)=w1377:u32)  [unwired: 1 out]
          }
          frame 6 {
            n662 = Split Number(x=w1387) -> (hi(x)=w1386:u32, lo(x)=w1385:u32)
          }
        }
        n663 = feedback-in #94(w1322) -> ()
        n664 = feedback-in #95(w1320) -> ()
        n665 = feedback-in #96(w1313) -> ()
        n666 = feedback-in #97(w1324) -> ()
        n667 = feedback-in #98(w1310) -> ()
      }
      frame 41 {
        n668 = call "_FPGA_MSProcess_ParameterHandler.vi"("Init"=w1399) -> ("Count"=w1398:u8, "U64 Data"=w1397:u64)  [unwired: 1 in]
        n669 = feedback #99() -> (w1395:bool)  [unwired: 1 in]
        n670 = case shown="1" w1398 {
          tunnel: w1397 -> [_ w1409 _]
          tunnel: [_ TRUE _] -> w1396
          tunnel: w1395 -> [_ _ w1410]
          frame 0, Default {
          }
          frame 1 {
            n671 = Split Number(x=w1409) -> (lo(x)=w1408:u32)  [unwired: 1 out]
            n672 = Split Number(x=w1408) -> (hi(x)=w1406:u16, lo(x)=w1407:u16)
            n673 = Split Number(x=w1406) -> (hi(x)=w1403:u8, lo(x)=w1405:u8)
            n674 = xnode ("Register Read")("Data"=w1405) -> ()  [unwired: 1 in, 1 out]
            n675 = xnode ("Register Write")("Data"=w1403) -> ()  [unwired: 1 in, 1 out]
            n676 = xnode ("Register Read")("Data"=w1407) -> ()  [unwired: 1 in, 1 out]
          }
          frame 2 {
            n677 = xnode ("Register Read")("Data"=w1410) -> ()  [unwired: 1 in, 1 out]
          }
        }
        n678 = feedback-in #99(w1396) -> ()
        n679 = xnode ("Register Write")() -> ("Data"=w1394:bool)  [unwired: 1 in, 1 out]
        n680 = call <instrlib>:"Detect Falling Edge.vi"("signal"=w1394) -> ("edge detected"=w1391:bool)  [unwired: 14 in]
        n681 = Select(t=u8 255, s=w1391, f=w1390) -> (s? t:f=w1393:u8)
      }
      frame 42 {
        n682 = call "_FPGA_MSProcess_ParameterHandler.vi"("Init"=w1415) -> ("Count"=w1414:u8, "U64 Data"=w1413:u64)  [unwired: 1 in]
        n683 = case shown="5" w1414 {
          tunnel: w1413 -> [_ w1428 w1437 w1446 w1455 _]
          tunnel: w1412 -> [w1419 w1422 w1431 w1440 w1449 _]
          tunnel: [w1419 w1422 w1431 w1440 w1449 u8 255] -> w1411
          frame 0, Default {
          }
          frame 1 {
            n684 = Split Number(x=w1428) -> (hi(x)=w1427:u32, lo(x)=w1420:u32)
            n685 = Split Number(x=w1427) -> (lo(x)=w1426:u16)  [unwired: 1 out]
            n686 = Split Number(x=w1426) -> (lo(x)=w1425:u8)  [unwired: 1 out]
            n687 = Number To Boolean Array(number=w1425) -> (Boolean array=w1424:bool[])
            n688 = Index Array(array=w1424, index=0) -> (element=w1421:bool)
            n689 = xnode ("Register Write")("Data"=w1420) -> ()  [unwired: 1 in, 1 out]
            n690 = xnode ("Register Write")("Data"=w1421) -> ()  [unwired: 1 in, 1 out]
          }
          frame 2 {
            n691 = Split Number(x=w1437) -> (hi(x)=w1436:u32, lo(x)=w1429:u32)
            n692 = Split Number(x=w1436) -> (lo(x)=w1435:u16)  [unwired: 1 out]
            n693 = Split Number(x=w1435) -> (lo(x)=w1434:u8)  [unwired: 1 out]
            n694 = Number To Boolean Array(number=w1434) -> (Boolean array=w1433:bool[])
            n695 = Index Array(array=w1433, index=0) -> (element=w1430:bool)
            n696 = xnode ("Register Write")("Data"=w1429) -> ()  [unwired: 1 in, 1 out]
            n697 = xnode ("Register Write")("Data"=w1430) -> ()  [unwired: 1 in, 1 out]
          }
          frame 3 {
            n698 = Split Number(x=w1446) -> (hi(x)=w1445:u32, lo(x)=w1438:u32)
            n699 = Split Number(x=w1445) -> (lo(x)=w1444:u16)  [unwired: 1 out]
            n700 = Split Number(x=w1444) -> (lo(x)=w1443:u8)  [unwired: 1 out]
            n701 = Number To Boolean Array(number=w1443) -> (Boolean array=w1442:bool[])
            n702 = Index Array(array=w1442, index=0) -> (element=w1439:bool)
            n703 = xnode ("Register Write")("Data"=w1438) -> ()  [unwired: 1 in, 1 out]
            n704 = xnode ("Register Write")("Data"=w1439) -> ()  [unwired: 1 in, 1 out]
          }
          frame 4 {
            n705 = Split Number(x=w1455) -> (hi(x)=w1454:u32, lo(x)=w1447:u32)
            n706 = Split Number(x=w1454) -> (lo(x)=w1453:u16)  [unwired: 1 out]
            n707 = Split Number(x=w1453) -> (lo(x)=w1452:u8)  [unwired: 1 out]
            n708 = Number To Boolean Array(number=w1452) -> (Boolean array=w1451:bool[])
            n709 = Index Array(array=w1451, index=0) -> (element=w1448:bool)
            n710 = xnode ("Register Write")("Data"=w1447) -> ()  [unwired: 1 in, 1 out]
            n711 = xnode ("Register Write")("Data"=w1448) -> ()  [unwired: 1 in, 1 out]
          }
          frame 5 {
          }
        }
      }
      frame 43 {
        n712 = call "_FPGA_MSProcess_ParameterHandler.vi"("Init"=w1461) -> ("Count"=w1460:u8, "U64 Data"=w1459:u64)  [unwired: 1 in]
        n713 = case shown="1" w1460 {
          tunnel: w1459 -> [_ w1470 _]
          tunnel: w1458 -> [w1465 w1466 _]
          tunnel: [w1465 w1466 u8 255] -> w1457
          frame 0, Default {
          }
          frame 1 {
            n714 = Split Number(x=w1470) -> (lo(x)=w1469:u32)  [unwired: 1 out]
            n715 = Split Number(x=w1469) -> (lo(x)=w1468:u16)  [unwired: 1 out]
            n716 = Split Number(x=w1468) -> (lo(x)=w1467:u8)  [unwired: 1 out]
            n717 = xnode ("Register Write")("Data"=w1467) -> ()  [unwired: 1 in, 1 out]
          }
          frame 2 {
          }
        }
      }
      frame 44 {
        n718 = call "_FPGA_MSProcess_ParameterHandler.vi"("Init"=w1476) -> ("Count"=w1475:u8, "U64 Data"=w1474:u64)  [unwired: 1 in]
        n719 = case shown="2" w1475 {
          tunnel: w1474 -> [_ w1499 _]
          tunnel: w1473 -> [w1480 w1496 _]
          tunnel: [w1480 w1496 u8 255] -> w1472
          frame 0, Default {
          }
          frame 1 {
            n720 = Split Number(x=w1499) -> (hi(x)=w1495:u32, lo(x)=w1498:u32)
            n721 = Split Number(x=w1495) -> (hi(x)=w1492:u16, lo(x)=w1493:u16)
            n722 = Split Number(x=w1498) -> (hi(x)=w1494:u16, lo(x)=w1497:u16)
            n723 = Split Number(x=w1492) -> (hi(x)=w1491:u8)  [unwired: 1 out]
            n724 = Split Number(x=w1493) -> (hi(x)=w1490:u8)  [unwired: 1 out]
            n725 = Split Number(x=w1494) -> (hi(x)=w1489:u8)  [unwired: 1 out]
            n726 = Split Number(x=w1497) -> (hi(x)=w1488:u8, lo(x)=w1487:u8)
            n727 = Number To Boolean Array(number=w1487) -> (Boolean array=w1486:bool[])
            n728 = Index Array(array=w1486, index #1=0 ("index")) -> (element #1=w1484:bool, element #2=w1483:bool, element #3=w1481:bool, element #4=w1482:bool)  [unwired: 3 in]
            n729 = xnode ("Register Write")("Data"=w1491) -> ()  [unwired: 1 in, 1 out]
            n730 = xnode ("Register Write")("Data"=w1489) -> ()  [unwired: 1 in, 1 out]
            n731 = xnode ("Register Write")("Data"=w1484) -> ()  [unwired: 1 in, 1 out]
            n732 = xnode ("Register Write")("Data"=w1481) -> ()  [unwired: 1 in, 1 out]
            n733 = xnode ("Register Write")("Data"=w1490) -> ()  [unwired: 1 in, 1 out]
            n734 = xnode ("Register Write")("Data"=w1488) -> ()  [unwired: 1 in, 1 out]
            n735 = xnode ("Register Write")("Data"=w1483) -> ()  [unwired: 1 in, 1 out]
            n736 = xnode ("Register Write")("Data"=w1482) -> ()  [unwired: 1 in, 1 out]
          }
          frame 2 {
          }
        }
      }
      frame 45 {
        n737 = call "_FPGA_MSProcess_ParameterHandler.vi"("Init"=w1505) -> ("Count"=w1504:u8, "U64 Data"=w1503:u64)  [unwired: 1 in]
        n738 = case shown="1" w1504 {
          tunnel: w1503 -> [_ w1514 _]
          tunnel: w1502 -> [w1509 w1513 _]
          tunnel: [w1509 w1513 u8 255] -> w1501
          frame 0, Default {
          }
          frame 1 {
            n739 = Split Number(x=w1514) -> (hi(x)=w1512:u32, lo(x)=w1511:u32)
            n740 = Split Number(x=w1512) -> (lo(x)=w1510:u16)  [unwired: 1 out]
            n741 = xnode ("Register Write")("Data"=w1511) -> ()  [unwired: 1 in, 1 out]
            n742 = xnode ("Register Write")("Data"=w1510) -> ()  [unwired: 1 in, 1 out]
          }
          frame 2 {
          }
        }
      }
    }
    n743 = feedback-in #35(w366) -> ()
    n744 = feedback-in #36(w364) -> ()
    n745 = feedback-in #37(w320) -> ()
    n746 = feedback-in #38(w371) -> ()
    n747 = feedback-in #40(w346) -> ()
    n748 = To Unsigned Quad Integer(1:w320) -> (0:w325:u64)
    n749 = xnode ("Register Read")() -> ("Data"=w277)  [unwired: 1 in, 1 out]
    n750 = xnode ("Register Read")() -> ("Data"=w365)  [unwired: 1 in, 1 out]
    n751 = xnode ("Register Read")() -> ("Data"=w288)  [unwired: 1 in, 1 out]
    n752 = xnode ("Register Read")() -> ("Data"=w278)  [unwired: 1 in, 1 out]
    n753 = xnode ("Register Read")() -> ("Data"=w269:u32)  [unwired: 1 in, 1 out]
    n754 = xnode ("Register Read")() -> ("Data"=w306:u64)  [unwired: 1 in, 1 out]
    n755 = xnode ("Register Read")() -> ("Data"=w372:bool)  [unwired: 1 in, 1 out]
    n756 = call "_FPGA_DDS_CycleAccumulator_version2.vi"("ConjSize"=w348, "Conj.InitCyc*2^32"=w349, "ConjArr"=w350, "Update_ConjArr_strobe"=w347, "DeCycle*2^32"=w325, "1/DeCyc*2^8"=w364, "Conj.Mode"=w288, "SlowCycle"=w365, "Reset"=w278, "IniCycle"=w277) -> ("LastConj_strobe?"=w303:bool, "Updating ConjArr?"=w360:bool, "Not Conj?"=w309:bool, "Conj Index"=w316:u8, "Cross Quadrant?"=w361:bool, "Quadrant"=w358:fxp<+,2,2>, "Cross Zero Phase?"=w357:bool, "RFCycleOut"=w287:u64)  [unwired: 2 in]
    n757 = feedback-in #28(w357) -> ()
    n758 = feedback-in #29(w358) -> ()
    n759 = feedback-in #30(w361) -> ()
    n760 = feedback-in #31(w316) -> ()
    n761 = feedback-in #32(w309) -> ()
    n762 = feedback-in #33(w360) -> ()
    n763 = feedback-in #34(w303) -> ()
    n764 = feedback-in #100(w287) -> ()
    n765 = feedback #100() -> (w308:u64)  [unwired: 1 in]
    n766 = feedback #101() -> (w293:u32)  [unwired: 1 in]
    n767 = feedback-in #101(w366) -> ()
    n768 = feedback #102() -> (w286:u64)  [unwired: 1 in]
    n769 = feedback-in #102(w287) -> ()
    n770 = feedback-in #103(w307) -> ()
    n771 = feedback #103() -> (w295:bool)  [unwired: 1 in]
    n772 = feedback #104() -> (w331:bool)  [unwired: 1 in]
    n773 = feedback-in #104(w332) -> ()
    n774 = xnode ("Register Read")() -> ("Data"=w273:u32)  [unwired: 1 in, 1 out]
    n775 = xnode ("Register Read")() -> ("Data"=w270:u32)  [unwired: 1 in, 1 out]
    n776 = xnode ("Register Read")() -> ("Data"=w335:u64)  [unwired: 1 in, 1 out]
    n777 = xnode ("Register Read")() -> ("Data"=w334:u64)  [unwired: 1 in, 1 out]
    n778 = feedback #105() -> (w315:u8)  [unwired: 1 in]
    n779 = feedback-in #105(w316) -> ()
    n780 = feedback #106() -> (w329:bool)  [unwired: 1 in]
    n781 = feedback-in #106(w309) -> ()
    n782 = xnode ("Register Read")() -> ("Data"=w342:u8)  [unwired: 1 in, 1 out]
    n783 = call "_FPGA_AuxPulseVoltageConvertor.vi"("Amp_in"=w270, "PulseBases_in"=w273) -> ("V Pulse 2"=w271:i16, "V Pulse 1"=w272:i16)  [unwired: 8 in]
    n784 = call "_FPGA_AuxCycCalculator.vi"("AuxIniCyc"=w306, "Init"=w295, "Scale*2^26"=w269, "PriRFCyc_U64"=w286) -> ("AuxCyc"=w281:u64)  [unwired: 7 in]
    n785 = feedback-in #39(w281) -> ()
    n786 = xnode ("Register Read")() -> ("Data"=w290)  [unwired: 1 in, 1 out]
    n787 = Number To Boolean Array(number=w342) -> (Boolean array=w341:bool[])
    n788 = Split Number(x=w308) -> (lo(x)=w294:u32)  [unwired: 1 out]
    n789 = Index Array(array=w341, index #1=1 ("index"), index #2=0 ("index")) -> (element #1=w336:bool, element #2=w339:bool)
    n790 = Split Number(x=w281) -> (lo(x)=w343:u32)  [unwired: 1 out]
    n791 = Equal To 0?(x=w315) -> (x = 0?=w314:bool)
    n792 = feedback #107() -> (w289)  [unwired: 1 in]
    n793 = feedback-in #107(w290) -> ()
    n794 = feedback #108() -> (w313:bool)  [unwired: 1 in]
    n795 = feedback-in #108(w314) -> ()
    n796 = feedback #109() -> (w312:bool)  [unwired: 1 in]
    n797 = feedback-in #109(w329) -> ()
    n798 = xnode ("Register Read")("Data"=w294) -> ()  [unwired: 1 in, 1 out]
    n799 = call "_FPGA_DigitalWfm_version2.vi"("Cycle in"=w294, "Amplitude*2^29"=w293) -> ("AuxVoltage"=w291:fxp<+/-,16,14>)  [unwired: 9 in]
    n800 = call "_FPGA_DDS_BMem_of_Cosine.vi"("Addr"=enum16{"Addr A", "Addr B"}."Addr A", "Cycle_in"=w294, "NormAmp*2^29"=w293) -> ("cos"=w292:fxp<+/-,16,14>)  [unwired: 8 in]
    n801 = call "_FPGA_Aux_ArbWfm.vi"("Cycle in"=w281) -> ("AuxVoltage"=w282:fxp<+/-,16,14>)  [unwired: 10 in]
    n802 = call "_FPGA_Aux_DigitalPulses.vi"("Cycle in"=w281, "reset"=w295, "TargetCycle2(i,f)"=w334, "AuxVoltage2"=w271, "TargetCycle1(i,f)"=w335, "AuxVoltage1"=w272) -> ("AuxVoltage"=w284:fxp<+/-,16,14>)  [unwired: 5 in]
    n803 = call "_FPGA_DigitalWfm_version2.vi"("Cycle in"=w343, "Amplitude*2^29"=w270) -> ("AuxVoltage"=w324:fxp<+/-,16,14>)  [unwired: 9 in]
    n804 = call "_FPGA_DDS_BMem_of_Cosine.vi"("Addr"=enum16{"Addr A", "Addr B"}."Addr B", "Cycle_in"=w343, "NormAmp*2^29"=w270) -> ("cos"=w337:fxp<+/-,16,14>)  [unwired: 8 in]
    n805 = feedback #110() -> (w296:bool)  [unwired: 1 in]
    n806 = feedback-in #110(w372) -> ()
    n807 = feedback #111() -> (w330:bool)  [unwired: 1 in]
    n808 = feedback-in #111(w331) -> ()
    n809 = Not(x=w312) -> (.not. x?=w310:bool)
    n810 = feedback-in #112(w336) -> ()
    n811 = feedback #112() -> (w304:bool)  [unwired: 1 in]
    n812 = feedback-in #113(w339) -> ()
    n813 = feedback #113() -> (w285:bool)  [unwired: 1 in]
    n814 = feedback #114() -> (w319:bool)  [unwired: 1 in]
    n815 = feedback-in #114(w312) -> ()
    n816 = feedback-in #115(w296) -> ()
    n817 = feedback #115() -> (w328:bool)  [unwired: 1 in]
    n818 = feedback #116() -> (w275:bool)  [unwired: 1 in]
    n819 = feedback-in #116(w330) -> ()
    n820 = And(x=w313, y=w310) -> (x .and. y?=w305:bool)
    n821 = Select(t=w282, s=w285, f=w284) -> (s? t:f=w283:fxp<+/-,16,14>)
    n822 = Select(t=w324, s=w285, f=w337) -> (s? t:f=w323:fxp<+/-,16,14>)
    n823 = Select(t=w283, s=w304, f=w323) -> (s? t:f=w322:fxp<+/-,16,14>)
    n824 = Select(t=w291, s=w289, f=w292) -> (s? t:f=w268:fxp<+/-,16,14>)
    n825 = Select(t=w322, s=w328, f=fxp<+/-,16,14> 0.0) -> (s? t:f=w280:fxp<+/-,16,14>)
    n826 = feedback #117() -> (w338:fxp<+/-,16,14>)  [unwired: 1 in]
    n827 = feedback-in #117(w280) -> ()
    n828 = feedback #118() -> (w276:bool)  [unwired: 1 in]
    n829 = feedback-in #118(w275) -> ()
    n830 = feedback-in #119(w268) -> ()
    n831 = feedback #119() -> (w344:fxp<+/-,16,14>)  [unwired: 1 in]
    n832 = Compound Arithmetic op=AND(invert w276, w275) -> (w274:bool)
    n833 = feedback #120() -> (w311:bool)  [unwired: 1 in]
    n834 = feedback-in #120(w305) -> ()
    n835 = feedback #121() -> (w326:bool)  [unwired: 1 in]
    n836 = feedback-in #121(w319) -> ()
    n837 = case shown="True" w274 {
      frame False {
      }
      frame True {
        n838 = xnode ("FIFO Method Node")("Element"=TRUE, "Timeout"=0) -> ()  [unwired: 1 in, 2 out]
      }
    }
    n839 = xnode ("Register Write")("Data"=w326) -> ()  [unwired: 1 in, 1 out]
    n840 = xnode ("FIFO Method Node")("Element"=w344, "Timeout"=0) -> ()  [unwired: 1 in, 2 out]
    n841 = xnode ("Register Write")("Data"=w311) -> ()  [unwired: 1 in, 1 out]
    n842 = xnode ("FIFO Method Node")("Element"=w338, "Timeout"=0) -> ()  [unwired: 1 in, 2 out]
    n843 = xnode ("FIFO Method Node")("Element"=w276, "Timeout"=0) -> ()  [unwired: 1 in, 2 out]
  }
  n844 = while {
    stop <- FALSE stop-if-true
    n845 = xnode ("Register Read")() -> ("Data"=→"SubEventCode":u8)  [unwired: 1 in, 1 out]
    n846 = xnode ("Register Write")() -> ("Data"=w1519:bool)  [unwired: 1 in, 1 out]
    n847 = xnode "FPGA I/O Node"("FPGA LED"=w1519) -> ()  [unwired: 1 in, 1 out]
  }
  n848 = node-c288() -> (w14:T3)  [unwired: 1 in]
  n849 = node-c288(w15) -> ()
  n850 = node-c288(w39) -> ()
  n851 = node-c288(w43) -> ()
  n852 = node-c288() -> (w32:T3)  [unwired: 1 in]
  n853 = timed-loop {
    timing: w14 -> [_]
    timing-out: [_] -> w13
    stop <- _ stop-if-true
    n854 = xnode ("Register Read")() -> ("Data"=w1555:u32)  [unwired: 1 in, 1 out]
    n855 = feedback #122(u32 0) -> (w1551:u32)
    n856 = Add(x=w1551, y=w1555) -> (x+y=w1552:u32)
    n857 = feedback-in #122(w1552) -> ()
    n858 = Split Number(x=w1551) -> (hi(x)=w1557:u16, lo(x)=w1546:u16)
    n859 = Split Number(x=w1557) -> (hi(x)=w1550:u8, lo(x)=w1549:u8)
    n860 = Increment(x=w1550) -> (x+1=w1556:u8)
    n861 = Join Numbers(hi=u8 0, lo=w1549) -> ((hi.lo)=w1547:u16)
    n862 = xnode ("Memory Method Node")("Address A"=w1556) -> ("Data A"=w1554:fxp<+/-,28,14>)  [unwired: 1 in, 1 out]
    n863 = xnode ("Memory Method Node")("Address B"=w1550) -> ("Data B"=w1553:fxp<+/-,28,14>)  [unwired: 1 in, 1 out]
    n864 = Join Numbers(hi=w1547, lo=w1546) -> ((hi.lo)=w1545:u32)
    n865 = feedback-in #123(w1545) -> ()
    n866 = feedback #123() -> (w1535:u32)  [unwired: 1 in]
    n867 = feedback-in #124(w1554) -> ()
    n868 = feedback #124() -> (w1532:fxp<+/-,28,14>)  [unwired: 1 in]
    n869 = feedback-in #125(w1553) -> ()
    n870 = feedback #125() -> (w1525:fxp<+/-,28,14>)  [unwired: 1 in]
    n871 = Subtract(x=w1532, y=w1525) -> (x-y=w1534:fxp<+/-,29,15>)
    n872 = To Fixed-Point(number=w1535) -> (fixed-point=w1544:fxp<+,24,24>)  [unwired: 1 in]
    n873 = To Fixed-Point(number=w1534) -> (fixed-point=w1533:fxp<+/-,23,9>)  [unwired: 1 in]
    n874 = xnode ("Register Read")() -> ("Data"=w1538:u16)  [unwired: 1 in, 1 out]
    n875 = Multiply(x=w1533, y=w1544) -> (x*y=w1543:fxp<+/-,47,33>)
    n876 = Scale By Power Of 2(n=i16 -24, x=w1543) -> (x*2^n=w1541:fxp<+/-,47,33>)
    n877 = Add(x=w1541, y=w1525) -> (x+y=w1536:fxp<+/-,48,34>)
    n878 = Round To Nearest(number=w1536) -> (nearest integer value=w1540:fxp<+/-,34,34>)
    n879 = feedback-in #126(w1538) -> ()
    n880 = feedback #126() -> (w1530:u16)  [unwired: 1 in]
    n881 = To Fixed-Point(fixed-point type=w1532, number=w1540) -> (fixed-point=w1539:fxp<+/-,28,14>)
    n882 = To Fixed-Point(number=w1530) -> (fixed-point=w1529:fxp<+,32,32>)  [unwired: 1 in]
    n883 = feedback-in #127(w1539) -> ()
    n884 = feedback #127() -> (w1531:fxp<+/-,28,14>)  [unwired: 1 in]
    n885 = Multiply(x=w1529, y=w1531) -> (x*y=w1528:fxp<+/-,60,46>)
    n886 = feedback-in #128(w1528) -> ()
    n887 = feedback #128() -> (w1527:fxp<+/-,60,46>)  [unwired: 1 in]
    n888 = Scale By Power Of 2(n=i16 -15, x=w1527) -> (x*2^n=w1521:fxp<+/-,60,46>)
    n889 = To Fixed-Point(fixed-point type=fxp<+/-,16,14> 0.0 ("Element"), number=w1521) -> (fixed-point=w1523:fxp<+/-,16,14>)
    n890 = feedback #129() -> (w1522:fxp<+/-,16,14>)  [unwired: 1 in]
    n891 = feedback-in #129(w1523) -> ()
    n892 = xnode ("FIFO Method Node")("Element"=w1522, "Timeout"=0) -> ()  [unwired: 1 in, 2 out]
  }
  n893 = timed-loop {
    timing: w32 -> [_]
    timing-out: [_] -> w31
    stop <- _ stop-if-true
    n894 = xnode ("Register Read")() -> ("Data"=w1574:u16)  [unwired: 1 in, 1 out]
    n895 = xnode ("Register Read")() -> ("Data"=w1561:u16)  [unwired: 1 in, 1 out]
    n896 = feedback #130() -> (w1562:bool)  [unwired: 1 in]
    n897 = Not(x=w1562) -> (.not. x?=w1563:bool)
    n898 = feedback-in #130(w1563) -> ()
    n899 = To Word Integer(number=w1561) -> (16bit integer=w1566:i16)
    n900 = call "_FPGA_Driver_FastADC.vi"("Clk_in"=w1562) -> ("Clk_out"=w1582:bool, "Output"=w1583:i16)  [unwired: 9 in]
    n901 = call "_FPGA_Timebase.vi"("HalfPeriod"=w1574) -> ("Clk_out"=w1585:bool)
    n902 = To Long Integer(number=w1583) -> (32bit integer=w1579:i32)
    n903 = feedback #131() -> (w1573:i16)  [unwired: 1 in]
    n904 = feedback-in #131(w1566) -> ()
    n905 = feedback #132() -> (w1580:i32)  [unwired: 1 in]
    n906 = feedback-in #132(w1579) -> ()
    n907 = feedback #133() -> (w1581:bool)  [unwired: 1 in]
    n908 = feedback-in #133(w1582) -> ()
    n909 = feedback-in #134(w1585) -> ()
    n910 = feedback #134() -> (w1576:bool)  [unwired: 1 in]
    n911 = call <instrlib>:"Detect Rising Edge.vi"("signal"=w1576) -> ("edge detected"=w1569:bool)  [unwired: 14 in]
    n912 = Negate(x=w1573) -> (-x=w1567:i16)
    n913 = Select(t=w1580, s=w1581, f=0) -> (s? t:f=w1578:i32)
    n914 = feedback #135() -> (w1577:i32)  [unwired: 1 in]
    n915 = Add(x=w1578, y=w1577) -> (x+y=w1568:i32)
    n916 = Scale By Power Of 2(n=w1567, x=w1568) -> (x*2^n=w1572:i32)
    n917 = Select(t=0 ("f"), s=w1569, f=w1568) -> (s? t:f=w1570:i32)
    n918 = feedback-in #135(w1570) -> ()
    n919 = To Word Integer(number=w1572) -> (16bit integer=w1564:i16)
    n920 = feedback #136() -> (w1584:i16)  [unwired: 1 in]
    n921 = feedback-in #136(w1564) -> ()
    n922 = feedback #137() -> (w1565:bool)  [unwired: 1 in]
    n923 = feedback-in #137(w1569) -> ()
    n924 = case shown="True" w1565 {
      tunnel: w1584 -> [_ w1586]
      frame False {
      }
      frame True {
        n925 = xnode ("FIFO Method Node")("Element"=w1586, "Timeout"=0) -> ()  [unwired: 1 in, 2 out]
      }
    }
  }
  n926 = node-c288() -> (w26:T3)  [unwired: 1 in]
  n927 = node-c288() -> (w24:T3)  [unwired: 1 in]
  n928 = node-c288() -> (w18:T3)  [unwired: 1 in]
  n929 = node-c288() -> (w30:T3)  [unwired: 1 in]
  n930 = timed-loop {
    timing: w26 -> [_]
    timing-out: [_] -> w25
    stop <- _ stop-if-true
    n931 = xnode ("Register Read")() -> ("Data"=w1591:u8)  [unwired: 1 in, 1 out]
    n932 = case shown="6" w1591 {
      tunnel: [w1592 w1593 w1594 w1595 w1596 w1597 w1598] -> w1590
      frame 0, Default {
        n933 = xnode ("Register Read")() -> ("Data"=w1592:bool)  [unwired: 1 in, 1 out]
      }
      frame 1 {
        n934 = xnode ("Register Read")() -> ("Data"=w1593:bool)  [unwired: 1 in, 1 out]
      }
      frame 2 {
        n935 = xnode ("Register Read")() -> ("Data"=w1594:bool)  [unwired: 1 in, 1 out]
      }
      frame 3 {
        n936 = xnode ("Register Read")() -> ("Data"=w1595:bool)  [unwired: 1 in, 1 out]
      }
      frame 4 {
        n937 = xnode ("Register Read")() -> ("Data"=w1596:bool)  [unwired: 1 in, 1 out]
      }
      frame 5 {
        n938 = xnode ("Register Read")() -> ("Data"=w1597:bool)  [unwired: 1 in, 1 out]
      }
      frame 6 {
        n939 = xnode ("Register Read")() -> ("Data"=w1598:bool)  [unwired: 1 in, 1 out]
      }
    }
    n940 = xnode "DO0"("DIO0"=w1590) -> ()  [unwired: 1 in, 1 out]
  }
  n941 = timed-loop {
    timing: w24 -> [_]
    timing-out: [_] -> w23
    stop <- _ stop-if-true
    n942 = xnode ("Register Read")() -> ("Data"=w1602:u8)  [unwired: 1 in, 1 out]
    n943 = case shown="6" w1602 {
      tunnel: [w1603 w1604 w1605 w1606 w1607 w1608 w1609] -> w1601
      frame 0, Default {
        n944 = xnode ("Register Read")() -> ("Data"=w1603:bool)  [unwired: 1 in, 1 out]
      }
      frame 1 {
        n945 = xnode ("Register Read")() -> ("Data"=w1604:bool)  [unwired: 1 in, 1 out]
      }
      frame 2 {
        n946 = xnode ("Register Read")() -> ("Data"=w1605:bool)  [unwired: 1 in, 1 out]
      }
      frame 3 {
        n947 = xnode ("Register Read")() -> ("Data"=w1606:bool)  [unwired: 1 in, 1 out]
      }
      frame 4 {
        n948 = xnode ("Register Read")() -> ("Data"=w1607:bool)  [unwired: 1 in, 1 out]
      }
      frame 5 {
        n949 = xnode ("Register Read")() -> ("Data"=w1608:bool)  [unwired: 1 in, 1 out]
      }
      frame 6 {
        n950 = xnode ("Register Read")() -> ("Data"=w1609:bool)  [unwired: 1 in, 1 out]
      }
    }
    n951 = xnode "DO1"("DIO1"=w1601) -> ()  [unwired: 1 in, 1 out]
  }
  n952 = timed-loop {
    timing: w18 -> [_]
    timing-out: [_] -> w17
    stop <- _ stop-if-true
    n953 = xnode ("FIFO Method Node")("Timeout"=0) -> ("Element"=w1617:fxp<+,14,14>, "Timed Out?"=w1616:bool)  [unwired: 1 in, 1 out]
    n954 = feedback #138() -> (w1618:fxp<+,14,14>)  [unwired: 1 in]
    n955 = Select(t=w1618, s=w1616, f=w1617) -> (s? t:f=w1615:fxp<+,14,14>)
    n956 = feedback-in #138(w1615) -> ()
    n957 = feedback #139() -> (w1612:bool)  [unwired: 1 in]
    n958 = Not(x=w1612) -> (.not. x?=w1613:bool)
    n959 = feedback-in #139(w1613) -> ()
    n960 = call "_FPGA_Driver_LTC1667_1_v1_3.vi"("Clk"=w1612, "Data in"=w1618) -> ()  [unwired: 10 in]
  }
  n961 = timed-loop {
    timing: w30 -> [_]
    timing-out: [_] -> w29
    stop <- _ stop-if-true
    n962 = xnode ("Register Read")() -> ("Data"=w1623:u8)  [unwired: 1 in, 1 out]
    n963 = call "_FPGA_Driver_V1.4DIO.vi"("DO"=w1623) -> ("DI"=w1622:u8)  [unwired: 10 in]
    n964 = xnode ("Register Write")("Data"=w1622) -> ()  [unwired: 1 in, 1 out]
    n965 = feedback-in #140(w1622) -> ()
    n966 = feedback #140() -> (→"DI":u8)  [unwired: 1 in]
  }
  n967 = node-c288(w27) -> ()
  n968 = node-c288(w25) -> ()
  n969 = node-c288(w23) -> ()
  n970 = node-c288() -> (w12:T3)  [unwired: 1 in]
  n971 = node-c288(w17) -> ()
  n972 = timed-loop {
    timing: w12 -> [_]
    timing-out: [_] -> w11
    stop <- _ stop-if-true
    n973 = xnode ("FIFO Method Node")("Timeout"=0) -> ("Element"=w1628, "Timed Out?"=w1630)  [unwired: 1 in, 1 out]
    n974 = feedback-in #141(w1628) -> ()
    n975 = feedback #141() -> (w1626)  [unwired: 1 in]
    n976 = feedback-in #142(w1630) -> ()
    n977 = feedback #142() -> (w1627)  [unwired: 1 in]
    n978 = case shown="False" w1627 {
      tunnel: w1626 -> [w1636 _]
      frame False {
        n979 = Split Number(x=w1636) -> (hi(x)=w1631:u16, lo(x)=w1635:u16)
        "AuxArbWfm" <- w1631
        n980 = Split Number(x=w1635) -> (lo(x)=w1634:u8)  [unwired: 1 out]
        n981 = Number To Boolean Array(number=w1634) -> (Boolean array=w1632:bool[])
        n982 = Boolean Array To Number(Boolean array=w1632) -> (number=w1633:fxp<+/-,9,9>)
        n983 = xnode ("Memory Method Node")("Address"=w1631, "Data"=w1633) -> ()  [unwired: 1 in, 1 out]
      }
      frame True {
      }
    }
  }
  n984 = node-c288(w37) -> ()
  n985 = node-c288(w29) -> ()
  n986 = node-c288() -> (w22:T3)  [unwired: 1 in]
  n987 = node-c288() -> (w20:T3)  [unwired: 1 in]
  n988 = node-c288() -> (w8:T3)  [unwired: 1 in]
  n989 = timed-loop {
    timing: w22 -> [_]
    timing-out: [_] -> w21
    stop <- _ stop-if-true
    n990 = xnode ("Register Read")() -> ("Data"=w1640:u8)  [unwired: 1 in, 1 out]
    n991 = case shown="0, Default" w1640 {
      tunnel: [w1641 w1642 w1643 w1644 w1645 w1646 w1647] -> w1639
      frame 0, Default {
        n992 = xnode ("Register Read")() -> ("Data"=w1641:bool)  [unwired: 1 in, 1 out]
      }
      frame 1 {
        n993 = xnode ("Register Read")() -> ("Data"=w1642:bool)  [unwired: 1 in, 1 out]
      }
      frame 2 {
        n994 = xnode ("Register Read")() -> ("Data"=w1643:bool)  [unwired: 1 in, 1 out]
      }
      frame 3 {
        n995 = xnode ("Register Read")() -> ("Data"=w1644:bool)  [unwired: 1 in, 1 out]
      }
      frame 4 {
        n996 = xnode ("Register Read")() -> ("Data"=w1645:bool)  [unwired: 1 in, 1 out]
      }
      frame 5 {
        n997 = xnode ("Register Read")() -> ("Data"=w1646:bool)  [unwired: 1 in, 1 out]
      }
      frame 6 {
        n998 = xnode ("Register Read")() -> ("Data"=w1647:bool)  [unwired: 1 in, 1 out]
      }
    }
    n999 = xnode "DO2"("DIO2"=w1639) -> ()  [unwired: 1 in, 1 out]
  }
  n1000 = timed-loop {
    timing: w20 -> [_]
    timing-out: [_] -> w19
    stop <- _ stop-if-true
    n1001 = xnode ("Register Read")() -> ("Data"=w1650:u8)  [unwired: 1 in, 1 out]
    n1002 = case shown="6" w1650 {
      tunnel: [w1652 w1653 w1654 w1655 w1656 w1657 w1658] -> w1651
      frame 0, Default {
        n1003 = xnode ("Register Read")() -> ("Data"=w1652:bool)  [unwired: 1 in, 1 out]
      }
      frame 1 {
        n1004 = xnode ("Register Read")() -> ("Data"=w1653:bool)  [unwired: 1 in, 1 out]
      }
      frame 2 {
        n1005 = xnode ("Register Read")() -> ("Data"=w1654:bool)  [unwired: 1 in, 1 out]
      }
      frame 3 {
        n1006 = xnode ("Register Read")() -> ("Data"=w1655:bool)  [unwired: 1 in, 1 out]
      }
      frame 4 {
        n1007 = xnode ("Register Read")() -> ("Data"=w1656:bool)  [unwired: 1 in, 1 out]
      }
      frame 5 {
        n1008 = xnode ("Register Read")() -> ("Data"=w1657:bool)  [unwired: 1 in, 1 out]
      }
      frame 6 {
        n1009 = xnode ("Register Read")() -> ("Data"=w1658:bool)  [unwired: 1 in, 1 out]
      }
    }
    n1010 = xnode "DO3"("DIO3"=w1651) -> ()  [unwired: 1 in, 1 out]
  }
  n1011 = timed-loop {
    timing: w8 -> [_]
    timing-out: [_] -> w7
    stop <- _ stop-if-true
    n1012 = xnode ("FIFO Method Node")("Timeout"=0) -> ("Element"=w1663:fxp<+,14,14>, "Timed Out?"=w1665:bool)  [unwired: 1 in, 1 out]
    n1013 = Not(x=w1665) -> (.not. x?=w1664:bool)
    n1014 = feedback-in #143(w1663, w1664) -> ()
    n1015 = feedback #143() -> (w1662:fxp<+,14,14>)  [unwired: 1 in]
    n1016 = feedback #144() -> (w1666:bool)  [unwired: 1 in]
    n1017 = Not(x=w1666) -> (.not. x?=w1667:bool)
    n1018 = feedback-in #144(w1667) -> ()
    n1019 = call "_FPGA_Driver_LTC1667_3_v1.3.vi"("Clk"=w1666, "Data_in"=w1662) -> ()  [unwired: 10 in]
  }
  n1020 = node-c288(w35) -> ()
  n1021 = node-c288(w31) -> ()
  n1022 = node-c288(w33) -> ()
  n1023 = node-c288(w7) -> ()
  n1024 = node-c288(w21) -> ()
  n1025 = node-c288(w19) -> ()
  n1026 = while {
    stop <- FALSE stop-if-true
    n1027 = xnode ("FIFO Method Node")() -> ("Number of Elements to Write"=→"SigI16 Ele#")  [unwired: 1 in, 1 out]
    n1028 = xnode ("FIFO Method Node")() -> ("Number of Elements to Read"=→"EventCode Ele#":u32)  [unwired: 1 in, 1 out]
    n1029 = xnode ("FIFO Method Node")() -> ("Number of Elements to Read"=→"RFU64 Ele#")  [unwired: 1 in, 1 out]
  }
  n1030 = node-c288(w13) -> ()
  n1031 = node-c288(w11) -> ()
  n1032 = node-c288(w41) -> ()
  n1033 = node-c288() -> (w10:T3)  [unwired: 1 in]
  n1034 = timed-loop {
    timing: w10 -> [_]
    timing-out: [_] -> w9
    stop <- _ stop-if-true
    w1721 = 0 ("Timeout")
    n1035 = xnode ("FIFO Method Node")("Timeout"=w1721) -> ("Element"=w1728:fxp<+/-,16,14>, "Timed Out?"=w1730:bool)  [unwired: 1 in, 1 out]
    n1036 = xnode ("FIFO Method Node")("Timeout"=w1721) -> ("Element"=w1723:fxp<+/-,16,14>, "Timed Out?"=w1722:bool)  [unwired: 1 in, 1 out]
    n1037 = xnode ("FIFO Method Node")("Timeout"=w1721) -> ("Element"=w1726:fxp<+/-,16,14>, "Timed Out?"=w1725:bool)  [unwired: 1 in, 1 out]
    n1038 = xnode ("Register Read")() -> ("Data"=w1719:fxp<+/-,16,14>)  [unwired: 1 in, 1 out]
    n1039 = xnode ("Register Read")() -> ("Data"=w1720:fxp<+/-,16,14>)  [unwired: 1 in, 1 out]
    n1040 = Not(x=w1730) -> (.not. x?=w1729:bool)
    n1041 = Not(x=w1725) -> (.not. x?=w1727:bool)
    n1042 = Not(x=w1722) -> (.not. x?=w1724:bool)
    n1043 = feedback-in #145(w1720) -> ()
    n1044 = feedback #145() -> (w1717:fxp<+/-,16,14>)  [unwired: 1 in]
    n1045 = feedback #146() -> (w1718:fxp<+/-,16,14>)  [unwired: 1 in]
    n1046 = feedback-in #146(w1728, w1729) -> ()
    n1047 = feedback #147() -> (w1716:fxp<+/-,16,14>)  [unwired: 1 in]
    n1048 = feedback-in #147(w1719) -> ()
    n1049 = feedback #148() -> (w1715:fxp<+/-,16,14>)  [unwired: 1 in]
    n1050 = feedback-in #148(w1726, w1727) -> ()
    n1051 = feedback #149() -> (w1692:fxp<+/-,16,14>)  [unwired: 1 in]
    n1052 = feedback-in #149(w1723, w1724) -> ()
    n1053 = Add "Aux"(x=w1717, y=w1718) -> (x+y=w1731:fxp<+/-,16,14>)
    n1054 = Add "Pri"(x=w1716, y=w1715) -> (x+y=w1694:fxp<+/-,16,14>)
    n1055 = Negate "OppAux"(x=w1731) -> (-x=w1699:fxp<+/-,16,14>)
    n1056 = Negate "OppPri"(x=w1694) -> (-x=w1693:fxp<+/-,16,14>)
    n1057 = Add "Pri+Aux"(x=w1731, y=w1694) -> (x+y=w1698:fxp<+/-,16,14>)
    n1058 = Add "Pri+OppAux"(x=w1699, y=w1694) -> (x+y=w1696:fxp<+/-,16,14>)
    n1059 = Add "OppPri+Aux"(x=w1731, y=w1693) -> (x+y=w1697:fxp<+/-,16,14>)
    n1060 = Add "OppPri+OppAux"(x=w1699, y=w1693) -> (x+y=w1695:fxp<+/-,16,14>)
    n1061 = xnode ("Register Read")() -> ("Data"=w1711:u8)  [unwired: 1 in, 1 out]
    n1062 = xnode ("Register Read")() -> ("Data"=w1706:u8)  [unwired: 1 in, 1 out]
    n1063 = xnode ("Register Read")() -> ("Data"=w1701:u8)  [unwired: 1 in, 1 out]
    n1064 = xnode ("Register Read")() -> ("Data"=w1682:fxp<+,32,32>)  [unwired: 1 in, 1 out]
    n1065 = xnode ("Register Read")() -> ("Data"=w1688:fxp<+,32,32>)  [unwired: 1 in, 1 out]
    n1066 = xnode ("Register Read")() -> ("Data"=w1676:fxp<+,32,32>)  [unwired: 1 in, 1 out]
    n1067 = xnode ("Register Read")() -> ("Data"=w1713:fxp<+/-,16,14>)  [unwired: 1 in, 1 out]
    n1068 = xnode ("Register Read")() -> ("Data"=w1708:fxp<+/-,16,14>)  [unwired: 1 in, 1 out]
    n1069 = xnode ("Register Read")() -> ("Data"=w1703:fxp<+/-,16,14>)  [unwired: 1 in, 1 out]
    n1070 = call "_FPGA_wfmMUX.vi"("OppAux"=w1699, "Aux"=w1731, "Sel"=w1711, "OppPri"=w1693, "Pri+Aux"=w1698, "OppPri+OppAux"=w1695, "FGEN"=w1692, "Pri+OppAux"=w1696, "OppPri+Aux"=w1697, "Pri"=w1694) -> ("SelectedWfm"=w1680:fxp<+/-,16,14>)  [unwired: 5 in]
    n1071 = call "_FPGA_wfmMUX.vi"("OppAux"=w1699, "Aux"=w1731, "Sel"=w1706, "OppPri"=w1693, "Pri+Aux"=w1698, "OppPri+OppAux"=w1695, "FGEN"=w1692, "Pri+OppAux"=w1696, "OppPri+Aux"=w1697, "Pri"=w1694) -> ("SelectedWfm"=w1686:fxp<+/-,16,14>)  [unwired: 5 in]
    n1072 = call "_FPGA_wfmMUX.vi"("OppAux"=w1699, "Aux"=w1731, "Sel"=w1701, "OppPri"=w1693, "Pri+Aux"=w1698, "OppPri+OppAux"=w1695, "FGEN"=w1692, "Pri+OppAux"=w1696, "OppPri+Aux"=w1697, "Pri"=w1694) -> ("SelectedWfm"=w1674:fxp<+/-,16,14>)  [unwired: 5 in]
    n1073 = Multiply(x=w1682, y=w1680) -> (x*y=w1684:fxp<+/-,48,46>)
    n1074 = Multiply(x=w1688, y=w1686) -> (x*y=w1690:fxp<+/-,48,46>)
    n1075 = Multiply(x=w1676, y=w1674) -> (x*y=w1678:fxp<+/-,48,46>)
    n1076 = Scale By Power Of 2(n=i16 -30, x=w1684) -> (x*2^n=w1685:fxp<+/-,48,46>)
    n1077 = Scale By Power Of 2(n=i16 -30, x=w1690) -> (x*2^n=w1689:fxp<+/-,48,46>)
    n1078 = Scale By Power Of 2(n=i16 -30, x=w1678) -> (x*2^n=w1679:fxp<+/-,48,46>)
    n1079 = To Fixed-Point(fixed-point type=w1680, number=w1685) -> (fixed-point=w1681:fxp<+/-,16,14>)
    n1080 = To Fixed-Point(fixed-point type=w1686, number=w1689) -> (fixed-point=w1687:fxp<+/-,16,14>)
    n1081 = To Fixed-Point(fixed-point type=w1674, number=w1679) -> (fixed-point=w1675:fxp<+/-,16,14>)
    n1082 = Add(x=w1681, y=w1713) -> (x+y=w1712:fxp<+/-,16,14>)
    n1083 = Add(x=w1687, y=w1708) -> (x+y=w1707:fxp<+/-,16,14>)
    n1084 = Add(x=w1675, y=w1703) -> (x+y=w1702:fxp<+/-,16,14>)
    n1085 = call "_FPGA_wfmFXPtoU14.vi"("wfmFXP"=w1707) -> ("U14"=w1709:fxp<+,14,14>)
    n1086 = call "_FPGA_wfmFXPtoU14.vi"("wfmFXP"=w1702) -> ("U14"=w1704:fxp<+,14,14>)
    n1087 = call "_FPGA_wfmFXPtoU14.vi"("wfmFXP"=w1712) -> ("U14"=w1714:fxp<+,14,14>)
    n1088 = xnode ("FIFO Method Node")("Element"=w1709, "Timeout"=0) -> ()  [unwired: 1 in, 2 out]
    n1089 = xnode ("FIFO Method Node")("Element"=w1704, "Timeout"=0) -> ()  [unwired: 1 in, 2 out]
    n1090 = xnode ("FIFO Method Node")("Element"=w1714, "Timeout"=0) -> ()  [unwired: 1 in, 2 out]
  }
  n1091 = node-c288(w9) -> ()
